vi "GUI_Beampointing2_Pico.vi"() -> ()   [LabVIEW 2013]
uses:
  shared programs/GUI_Template/GUI_master/tcp_new_data_event.ctl
  shared programs/GUI_Template/GUI_master/tcp new data cluster.ctl
  Ctrs/beam detection.ctl
  Ctrs/move_old.ctl
  Ctrs/stats.ctl
  Ctrs/Motor Calibration.ctl
  <vilib>/Analysis/NI_AALBase.lvlib
panel:
  in  "size 2":cluster{"xhair size":dbl, "xhair size 2":dbl}={"xhair size"=20.0, "xhair size 2"=20.0} {"xhair size 2" min=0.0 max=0.0; "xhair size" min=0.0 max=0.0}
  in  "Time":timestamp[](array[timestamp])
  in  "Stats 2":T1
  in  "output cluster 2":T2
  in  "UDP error message":string
  in  "Save Stats":bool
  in  "output cluster":T6={"img to avg"=0, "beam detection para"={"Filter"=0, "Filter Para"={"X Size"=0, "Y Size"=0, "% Tolerance"=0}, "detection method"=0, "smal para"=[], "Remove small Objects"=FALSE, "Restrict to round Objects"=FALSE}, "move"={"Tolerance [%]"=0.1, "Stepsize"=0.0001, "Invert Axis"=TRUE, "Invert Direction X"=FALSE, "Invert Direction Y"=TRUE, "enable feedback"=FALSE, "Set Centriod Target"=FALSE, "my active motor"=""}, "GUIdevice 1"="", "GUIdevice 2"="", "ActiveMotor"=0, "stats path "=path ""} {"beam detection para"."smal para"."Measurement Parameter" items=["Center of Mass X", "Center of Mass Y", "First Pixel X", "First Pixel Y", "Bounding Rect Left", "Bounding Rect Top", "Bounding Rect Right", "Bounding Rect Bottom", "Max Feret Diameter Start X", "Max Feret Diameter Start Y", "Max Feret Diameter End X", "Max Feret Diameter End Y", "Max Horiz. Segment Length Left", "Max Horiz. Segment Length Right", "Max Horiz. Segment Length Row", "-", "Bounding Rect Width", "Bounding Rect Height", "Bounding Rect Diagonal", "Perimeter", "Convex Hull Perimeter", "Holes' Perimeter", "Max Feret Diameter", "Equivalent Ellipse Major Axis", "Equivalent Ellipse Minor Axis", "Equivalent Ellipse Minor Axis (Feret)", "Equivalent Rect Long Side", "Equivalent Rect Short Side", "Equivalent Rect Diagonal", "Equivalent Rect Short Side (Feret)", "Average Horiz. Segment Length", "Average Vert. Segment Length", "Hydraulic Radius", "Waddel Disk Diameter", "-", "Area", "Holes' Area", "Particle & Holes' Area", "Convex Hull Area", "Image Area", "-", "Number of Holes", "Number of Horiz. Segments", "Number of Vert. Segments", "-", "Orientation", "Max Feret Diameter Orientation", "-", "% Area/Image Area", "% Area/(Particle & Holes' Area)", "Ratio of Equivalent Ellipse Axes", "Ratio of Equivalent Rect Sides", "-", "Elongation Factor", "Compactness Factor", "Heywood Circularity Factor", "Type Factor", "-", "Sum X", "Sum Y", "Sum XX", "Sum XY", "Sum YY", "Sum XXX", "Sum XXY", "Sum XYY", "Sum YYY", "-", "Moment of Inertia XX", "Moment of Inertia XY", "Moment of Inertia YY", "Moment of Inertia XXX", "Moment of Inertia XXY", "Moment of Inertia XYY", "Moment of Inertia YYY", "Norm. Moment of Inertia XX", "Norm. Moment of Inertia XY", "Norm. Moment of Inertia YY", "Norm. Moment of Inertia XXX", "Norm. Moment of Inertia XXY", "Norm. Moment of Inertia XYY", "Norm. Moment of Inertia YYY", "Hu Moment 1", "Hu Moment 2", "Hu Moment 3", "Hu Moment 4", "Hu Moment 5", "Hu Moment 6", "Hu Moment 7"]; "beam detection para"."smal para"."Range Lower Value" format="%.2f"; "beam detection para"."smal para"."Range Upper Value" format="%.2f"; "beam detection para"."detection method" items=["clustering", "entropy", "metric", "moments", "inter-class variance"]; "beam detection para"."Filter" items=["No Filter", "Median Filter", "Low Pass Filter"]}
  in  "Trigger::1":bool
  in  "Triggerdelay::1":dbl=0.003 min=0.0 max=0.09 format="%#_6f"
  in  "Exposure::1":dbl=0.095 min=0.0001 max=1.0 format="%#_6f"
  in  "ActiveMotorName::2":string
  in  "RelativeSettings.Axis 1.StepSize::2":dbl=50.0 caption="Axis 1 Stepsize" min=0.0 max=999999.0 format="%_4p"
  in  "RelativeSettings.Axis 2.StepSize::2":dbl=50.0 caption="Axis 2 StepSize" min=0.0 max=999999.0 format="%_4p"
  in  "RelativeSettings.Axis 2.Position::2":dbl caption="Axis 2 Position" min=-999999.0 max=999999.0 format="%_4p"
  in  "RelativeSettings.Axis 1.Position::2":dbl caption="Axis 1 Position" min=-999999.0 max=999999.0 format="%_4p"
  in  "RelativeMove.Axis 2.CW::2":bool caption="RelativeMove.Axis 2.CW::1"
  in  "RelativeMove.Axis 2.CCW::2":bool caption="RelativeMove.Axis. 2.CCW::1"
  in  "RelativeMove.Axis 1.CW::2":bool caption="RelativeMove.Axis 1.CW::1"
  in  "RelativeMove.Axis 1.CCW::2":bool caption="RelativeMove.Axis 1.CCW::1"
  out "Names":string[](array[string])=["PA2_Input1", "PA2_Input2", "L2_TelInpFar", "L1_TelInpNear", "L4_TREXPASS1", "L5_TREXPass2", "L6_TREXPass3", "L7_TREXPass4", "L8_M10Leak", "B1_TelInput", "B2_TelLens1"]
  in  "ActiveMotor":u16(ring)=7
  in  "Set Centriod Target":bool
  in  "size":dbl=10.299999999999997
  in  "Tab Control 2":enum32{"CCD Original ", "CCD Detected"}(tab)=enum."CCD Detected"
  out "image::1":T7(plugin-control) caption="StagingM1Far"
  out "Beam":T7(plugin-control)
  in  "Reset History":bool
  out "centriod X":dbl[](graph)=[249.59745762711864, 249.9873417721519, 249.85593220338984]
  out "centriod Y":dbl[](graph)=[256.39830508474574, 256.0126582278481, 257.0]
  out "Stats":cluster{timestamp[], dbl[]}[](graph)
  in  "Tab Control":enum32{"System", "Detection", "Feedback"}(tab)=enum."Feedback"
  in  "Save Stats":bool
  in  "update speed [ms]":i32=200
  in  "img to avg":i32=20
  in  "Save Config":bool
  in  "Load Config":bool
  in  "Cameras":u16(ring)=15 items=["10TW_Driver_Spot_Cam", "B1_TelInput", "B2_TelLens1", "B3_TelLens2", "B5_CompressorOut", "B6_SwitchYNear", "B9_OAPFront", "GIGEtest", "L1_TelInpNear", "L2_TelInpFar", "L3_TelescopeOut", "L4_TREXpass1", "L5_TREXPass2", "L6_TREXpass3", "L7_TREXPass4", "L8_M10Leak", "OAPtestCam", "PA2_Input1", "PA2_Input2", "PaperCam", "StagingAlignBeam1", "StagingAlignBeam2", "StagingCapAlignment", "StagingCapSpec", "StagingCapSpec1stOrder", "StagingChromaxGuppy", "StagingDiodeMonitor", "StagingFocusBeam1", "StagingFocusBeam2", "StagingGuppy", "StagingM1Far", "StagingM1Near", "StagingM3Far", "StagingM4", "StagingM5", "StagingMagnetCam1", "StagingMagnetCam2", "StagingMagnetCam3", "StagingManta2", "StagingModeImager2", "StagingModeTemp", "StagingOAP1Far", "StagingOAP1Near", "StagingOAP2Far", "StagingOAP2Near", "StagingPhasics", "StagingPhosphor", "StagingTapeCam", "StagingTapeMonitorCam", "StagingTopView", "TargetCam10Hz_Diode", "TargetCam1Hz_Pulsed", "TREXVarianCam0", "TREXVarianCam1", "TREXVarianCam2", "TREXVarianCam3", "TREX_CapSideView", "TREX_TA6", "TS-253a_in", "TS-CapSideview", "TS-CapSpec", "TS-ChromexCam", "TS-InputNearField", "TS-Mode1", "TS-OverlapCam", "TS-Periscope", "XUV_Cam1", "XUV_Cam2"]
  in  "calibrate":bool
  in  "stats path":path
  in  "beam detection para":T3={"Filter"=1, "Filter Para"={"X Size"=5, "Y Size"=5, "% Tolerance"=1}, "detection method"=4, "smal para"=[{"Measurement Parameter"=35, "Range Lower Value"=150.0, "Range Upper Value"=300.0, "Range"=FALSE, "Measurement Type"=FALSE}], "Remove small Objects"=TRUE, "Restrict to round Objects"=FALSE} {"smal para"."Measurement Parameter" items=["Center of Mass X", "Center of Mass Y", "First Pixel X", "First Pixel Y", "Bounding Rect Left", "Bounding Rect Top", "Bounding Rect Right", "Bounding Rect Bottom", "Max Feret Diameter Start X", "Max Feret Diameter Start Y", "Max Feret Diameter End X", "Max Feret Diameter End Y", "Max Horiz. Segment Length Left", "Max Horiz. Segment Length Right", "Max Horiz. Segment Length Row", "-", "Bounding Rect Width", "Bounding Rect Height", "Bounding Rect Diagonal", "Perimeter", "Convex Hull Perimeter", "Holes' Perimeter", "Max Feret Diameter", "Equivalent Ellipse Major Axis", "Equivalent Ellipse Minor Axis", "Equivalent Ellipse Minor Axis (Feret)", "Equivalent Rect Long Side", "Equivalent Rect Short Side", "Equivalent Rect Diagonal", "Equivalent Rect Short Side (Feret)", "Average Horiz. Segment Length", "Average Vert. Segment Length", "Hydraulic Radius", "Waddel Disk Diameter", "-", "Area", "Holes' Area", "Particle & Holes' Area", "Convex Hull Area", "Image Area", "-", "Number of Holes", "Number of Horiz. Segments", "Number of Vert. Segments", "-", "Orientation", "Max Feret Diameter Orientation", "-", "% Area/Image Area", "% Area/(Particle & Holes' Area)", "Ratio of Equivalent Ellipse Axes", "Ratio of Equivalent Rect Sides", "-", "Elongation Factor", "Compactness Factor", "Heywood Circularity Factor", "Type Factor", "-", "Sum X", "Sum Y", "Sum XX", "Sum XY", "Sum YY", "Sum XXX", "Sum XXY", "Sum XYY", "Sum YYY", "-", "Moment of Inertia XX", "Moment of Inertia XY", "Moment of Inertia YY", "Moment of Inertia XXX", "Moment of Inertia XXY", "Moment of Inertia XYY", "Moment of Inertia YYY", "Norm. Moment of Inertia XX", "Norm. Moment of Inertia XY", "Norm. Moment of Inertia YY", "Norm. Moment of Inertia XXX", "Norm. Moment of Inertia XXY", "Norm. Moment of Inertia XYY", "Norm. Moment of Inertia YYY", "Hu Moment 1", "Hu Moment 2", "Hu Moment 3", "Hu Moment 4", "Hu Moment 5", "Hu Moment 6", "Hu Moment 7"]; "smal para"."Range Lower Value" format="%.2f"; "smal para"."Range Upper Value" format="%.2f"; "detection method" items=["clustering", "entropy", "metric", "moments", "inter-class variance"]; "Filter" items=["No Filter", "Median Filter", "Low Pass Filter"]}
  in  "Move Properties":T5={"Tolerance [%]"=0.1, "Stepsize"=0.0001, "Invert Axis"=TRUE, "Invert Direction X"=FALSE, "Invert Direction Y"=TRUE, "enable feedback"=FALSE, "Set Centriod Target"=FALSE, "my active motor"=""} {"Stepsize" format="%#_6p"}
  out "Y Size":dbl=20.599999999999994
  out "X Size":dbl=15.599999999999994
  out "Particle Reports (Pixels)":T8(array[cluster])=[{"Area"=236.0, "Number of Holes"=0.0, "Bounding Rect"={"Left"=243.0, "Top"=247.0, "Right"=258.0, "Bottom"=268.0}, "Center of Mass"={"X"=249.85593220338984, "Y"=257.0}, "Orientation"=87.89795034558499, "Dimensions"={"Width"=15.0, "Height"=21.0}}] {"Orientation" format="%.2f"; "Dimensions"."Height" format="%.2f"; "Dimensions"."Width" format="%.2f"; "Center of Mass"."Y" format="%.2f"; "Center of Mass"."X" format="%.2f"; "Bounding Rect"."Bottom" format="%.2f"; "Bounding Rect"."Right" format="%.2f"; "Bounding Rect"."Top" format="%.2f"; "Bounding Rect"."Left" format="%.2f"; "Number of Holes" format="%.2f"; "Area" format="%.2f"}
  out "move required":bool=TRUE
  out "moving":bool
  out "Best Rectangle":T9(array[cluster])=[{"Left"=243.0, "Top"=247.0, "Right"=259.0, "Bottom"=267.0}, {"Left"=242.0, "Top"=246.0, "Right"=257.0, "Bottom"=267.0}, {"Left"=242.0, "Top"=246.0, "Right"=258.0, "Bottom"=267.0}, {"Left"=243.0, "Top"=247.0, "Right"=258.0, "Bottom"=268.0}, {"Left"=242.0, "Top"=247.0, "Right"=258.0, "Bottom"=267.0}]
  out "XY Graph":cluster{timestamp[], dbl[]}[](graph)
  out "Y offset":dbl=-1.5635377104373447
  out "X offset":dbl=10.405838585398385
  in  "Target.X::1":dbl=260.0 min=0.0 max=2000.0 format="%#_6f"
  in  "Target.Y::1":dbl=255.0 min=0.0 max=2000.0 format="%#_6f"
  out "mean Y":dbl=256.56353771043734 format="%0.2f"
  out "mean X":dbl=249.59416141460161 format="%0.2f"
  out "beam detected":bool=TRUE
  in  "GUIdevice 2":string="Picopad4"
  out "error out":errorcluster
  in  "insert tag":bool=TRUE
  in  "stop":bool=TRUE
  in  "GUIdevice 1":string="B5_CompressorOut"
  out "tcp data event":T10
  out "error IO 2":errorcluster
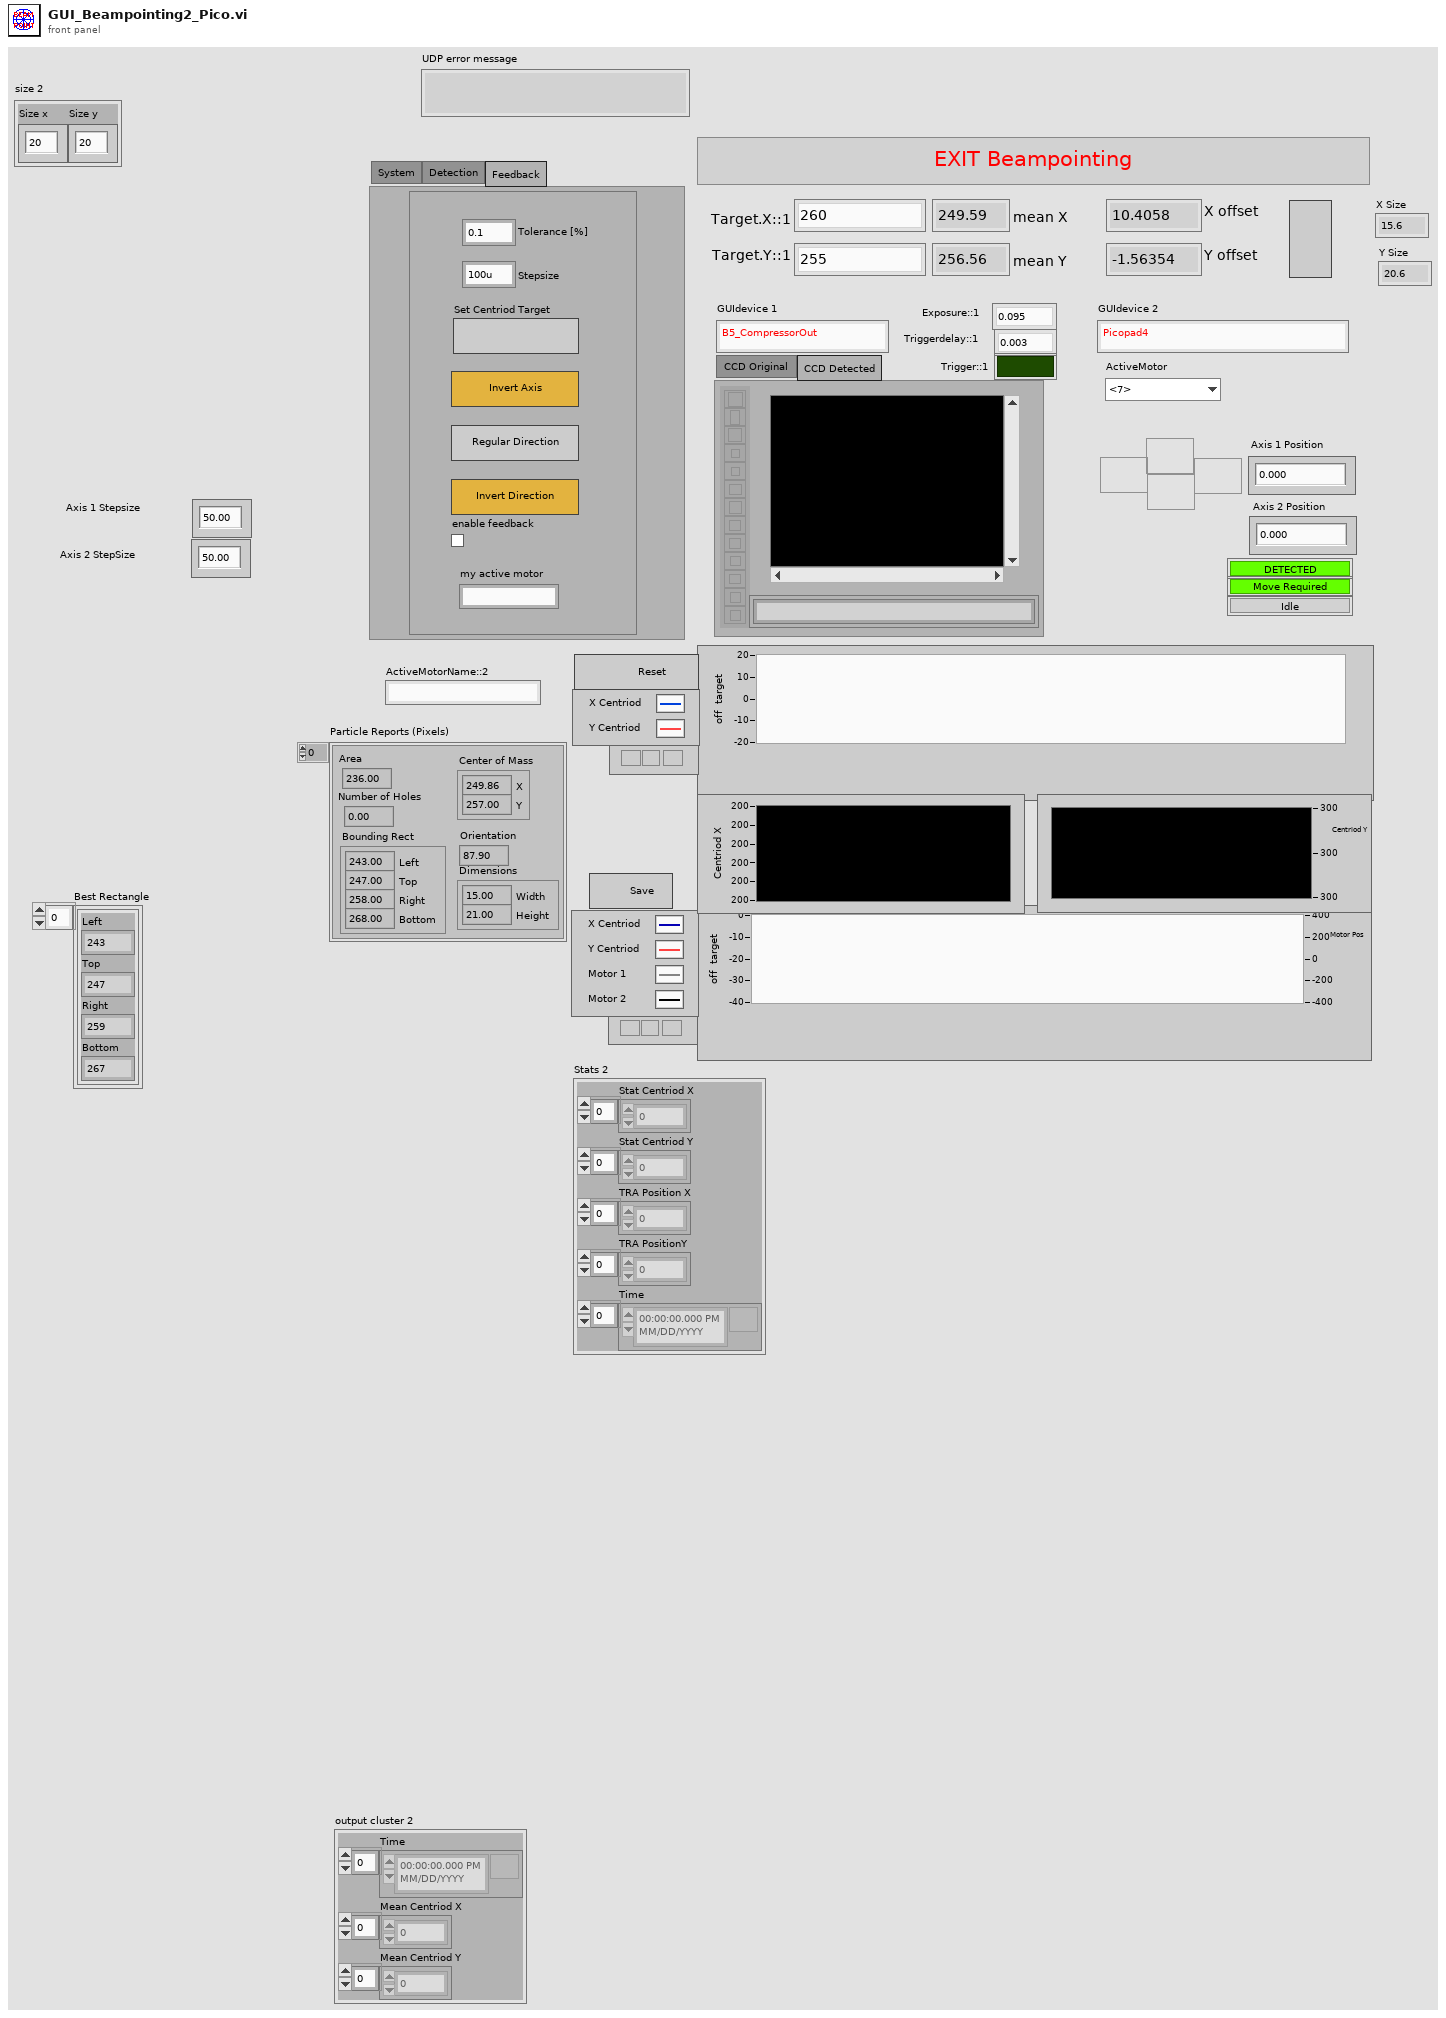
[diagram p1: front panel]
types:
  T1 = typedef "stats.ctl" = cluster{"Stat Centriod X":dbl[], "Stat Centriod Y":dbl[], "TRA Position X":dbl[], "TRA PositionY":dbl[], "Time":timestamp[]}
  T2 = cluster{"Time":timestamp[], "Mean Centriod X":dbl[], "Mean Centriod Y":dbl[]}
  T3 = typedef "beam detection.ctl" = cluster{"Filter":u16, "Filter Para":cluster{"X Size":i32, "Y Size":i32, "% Tolerance":i32}, "detection method":i32, "smal para":cluster{"Measurement Parameter":T4, "Range Lower Value":dbl, "Range Upper Value":dbl, "Range":bool, "Measurement Type":bool}[], "Remove small Objects":bool, "Restrict to round Objects":bool}
  T4 = typedef "Particle Parameters" = i32
  T5 = typedef "move_old.ctl" = cluster{"Tolerance [%]":dbl, "Stepsize":dbl, "Invert Axis":bool, "Invert Direction X":bool, "Invert Direction Y":bool, "enable feedback":bool, "Set Centriod Target":bool, "my active motor":string}
  T6 = cluster{"img to avg":i32, "beam detection para":T3, "move":T5, "GUIdevice 1":string, "GUIdevice 2":string, "ActiveMotor":u16, "stats path ":path}
  T7 = typedef "IMAQ Image.ctl" = refnum<image>
  T8 = cluster{"Area":dbl, "Number of Holes":dbl, "Bounding Rect":cluster{"Left":dbl, "Top":dbl, "Right":dbl, "Bottom":dbl}, "Center of Mass":cluster{"X":dbl, "Y":dbl}, "Orientation":dbl, "Dimensions":cluster{"Width":dbl, "Height":dbl}}[]
  T9 = cluster{"Left":dbl, "Top":dbl, "Right":dbl, "Bottom":dbl}[]
  T10 = typedef "tcp_new_data_event.ctl" = refnum<user-event>
  T11 = typedef "tcp new data cluster.ctl" = cluster{"EventEnum":enum16{"new data", "connection status update"}, "Device name":string}
  T12 = typedef "Image Type" = u32
  T13 = cluster{"RelativeMove.Axis 1.CW::2":refnum<vi>, "RelativeMove.Axis 1.CCW::2":refnum<vi>, "RelativeMove.Axis 2.CW::2":refnum<vi>, "RelativeMove.Axis 2.CCW::2":refnum<vi>}
  T14 = cluster{"Left":i32, "Top":i32, "Right":i32, "Bottom":i32}
  T15 = enum32{"invalid app kind", "Development System", "Run Time System", "Student Edition", "Embedded LabVIEW", "Evaluation", "Custom"}
  T16 = enum32{"Invalid", "Standard", "Closed", "Hidden", "Minimized", "Maximized"}
  T17 = enum16{"open", "replace", "create", "open or create", "replace or create", "replace or create with confirmation"}
  T18 = typedef "Motor Calibration.ctl" = cluster{"Slope Axis 1":dbl, "Axis Inverted":bool, "Slope Axis 2":dbl, "Axis 1 revered":bool, "Axis 2 revered":bool}
  T19 = cluster{"Core":cluster{"Current VI Reference":refnum<vi>, "Close Panel on Exit?":bool}, "beam detection para":T3, "Centriod X":dbl[], "Centriod Y":dbl[], "Best Rectangle":cluster{"Left":dbl, "Top":dbl, "Right":dbl, "Bottom":dbl}[], "PArticle Report":cluster{"Area":dbl, "Number of Holes":dbl, "Bounding Rect":cluster{"Left":dbl, "Top":dbl, "Right":dbl, "Bottom":dbl}, "Center of Mass":cluster{"X":dbl, "Y":dbl}, "Orientation":dbl, "Dimensions":cluster{"Width":dbl, "Height":dbl}}[], "Mean Centriod X":dbl[], "Mean Centriod Y":dbl[], "Time":timestamp[], "beam detected":bool, "offsets":cluster{"X offset":dbl, "Y offset":dbl}, "move":T5, "moving":bool, "Stats":T1, "set centriod target":bool, "Motor Calibration":T18}
  T20 = cluster{"Left":dbl, "Top":dbl, "Right":dbl, "Bottom":dbl}
  T21 = cluster{"Current VI Reference":refnum<vi>, "Close Panel on Exit?":bool}
  T22 = cluster{"Time":timestamp[], "Stat Centriod X":dbl[]}
  T23 = cluster{"Time":timestamp[], "Stat Centriod Y":dbl[]}
  T24 = cluster{"Time":timestamp[], "TRA Position X":dbl[]}
  T25 = cluster{"Time":timestamp[], "TRA PositionY":dbl[]}
  T26 = cluster{"Time":timestamp[], "TRA PositionY":dbl[]}[]
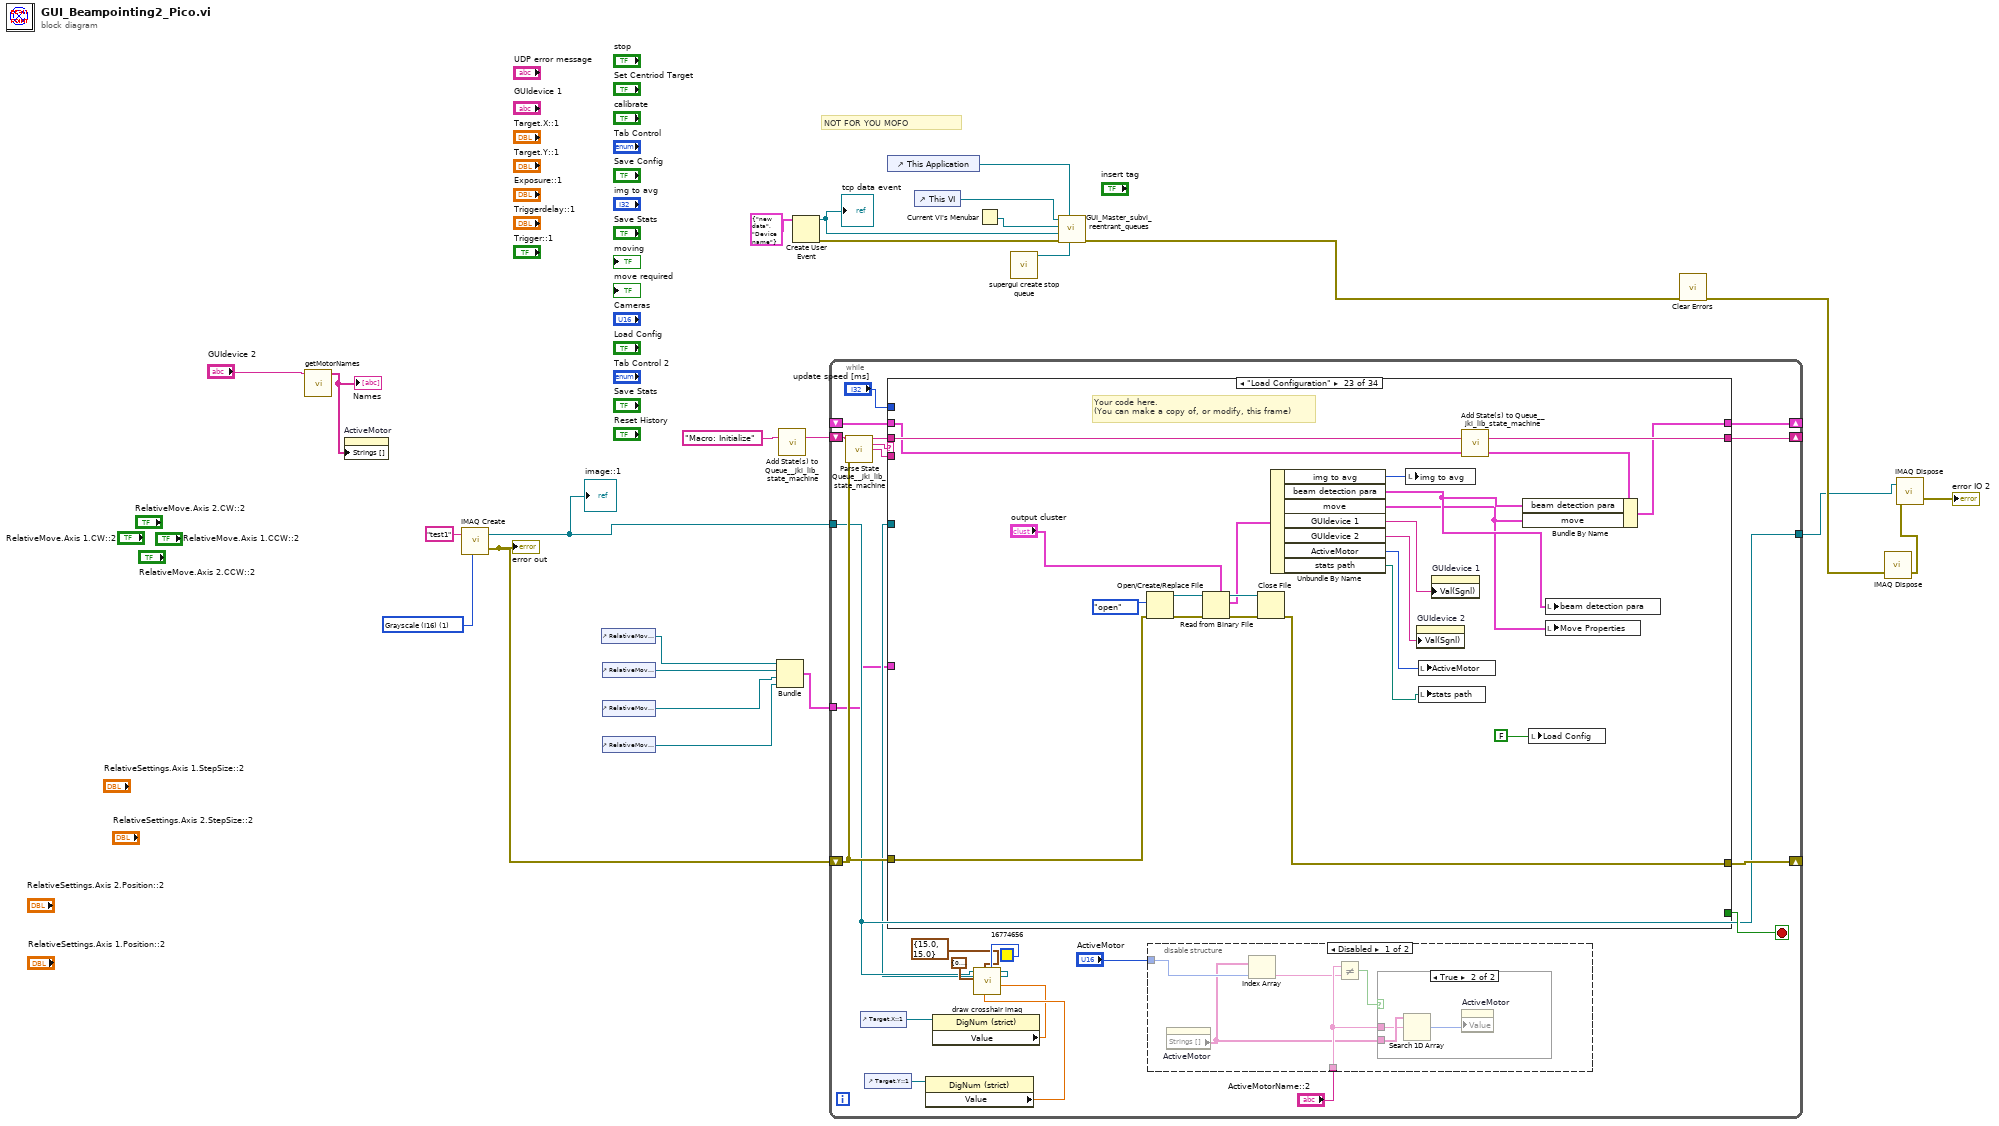
[diagram p0: block diagram]
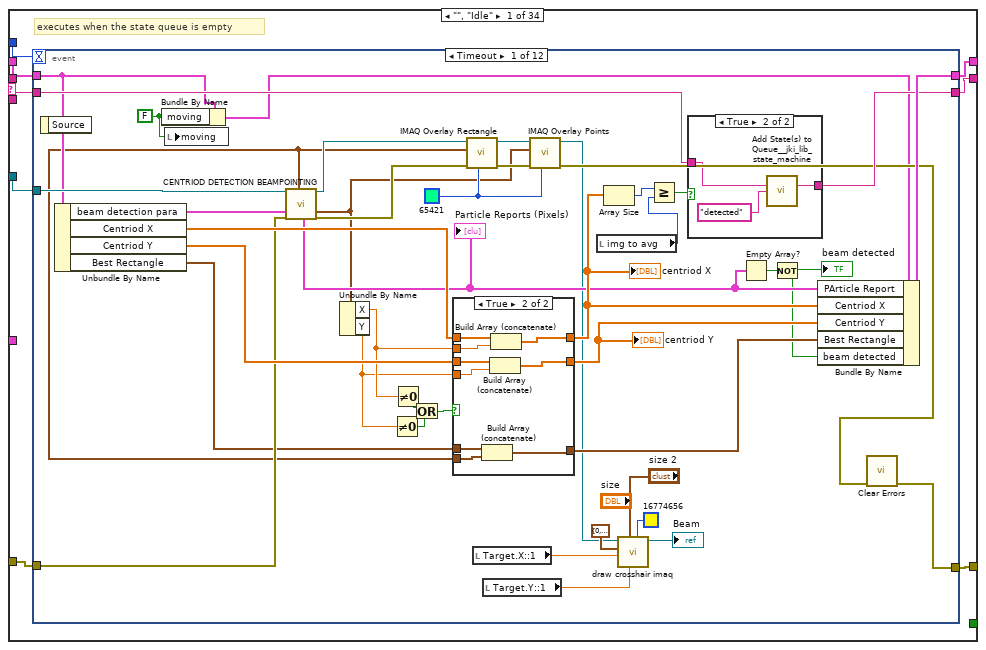
[diagram p4: hidden frame]
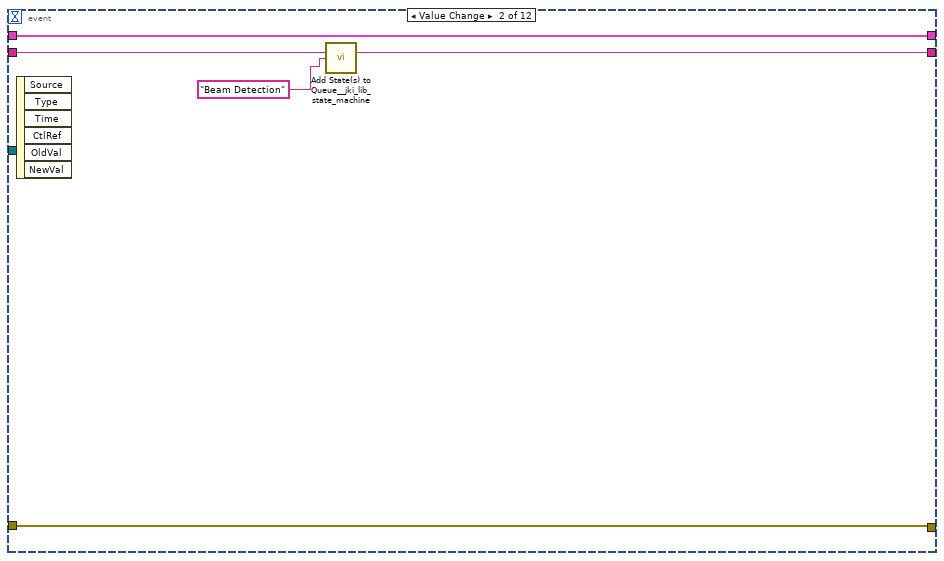
[diagram p7: hidden frame]
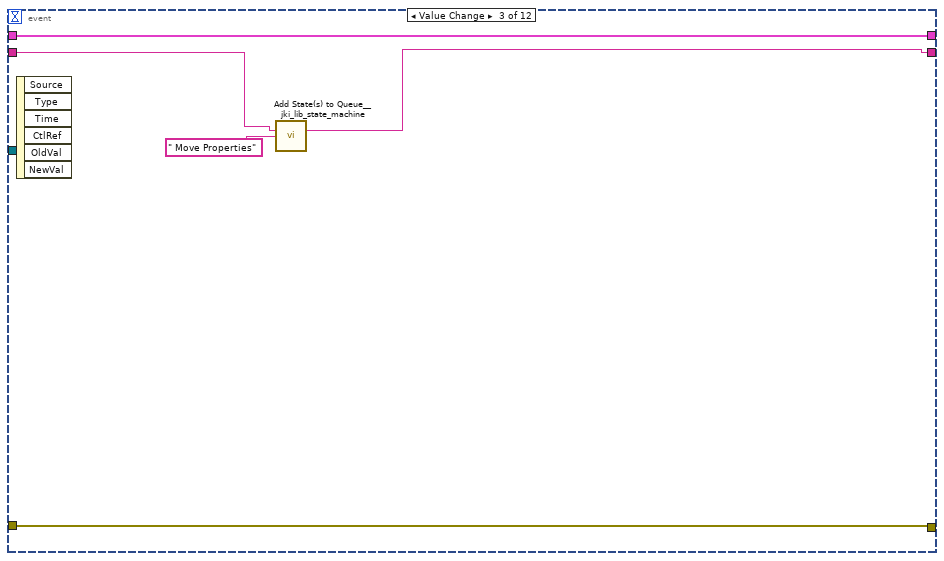
[diagram p8: hidden frame]
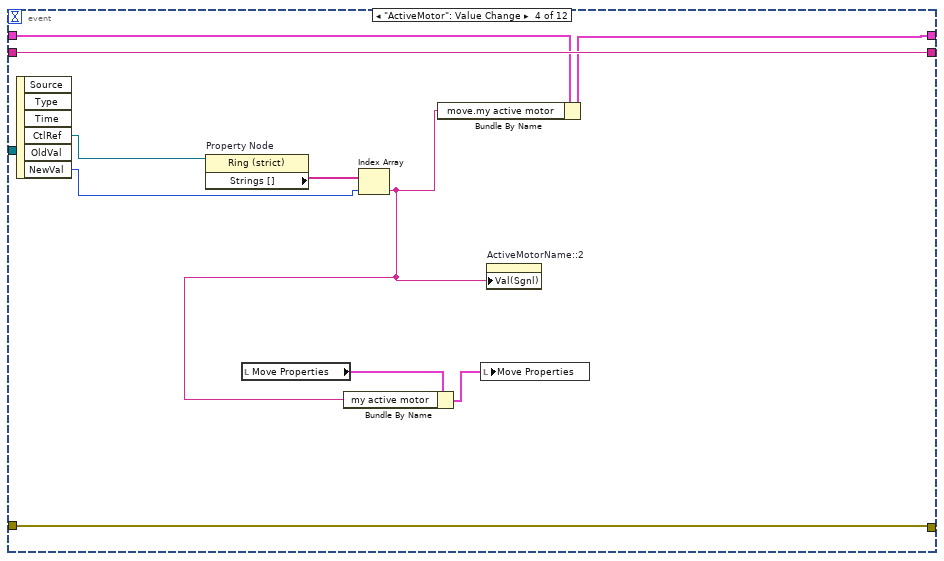
[diagram p9: hidden frame]
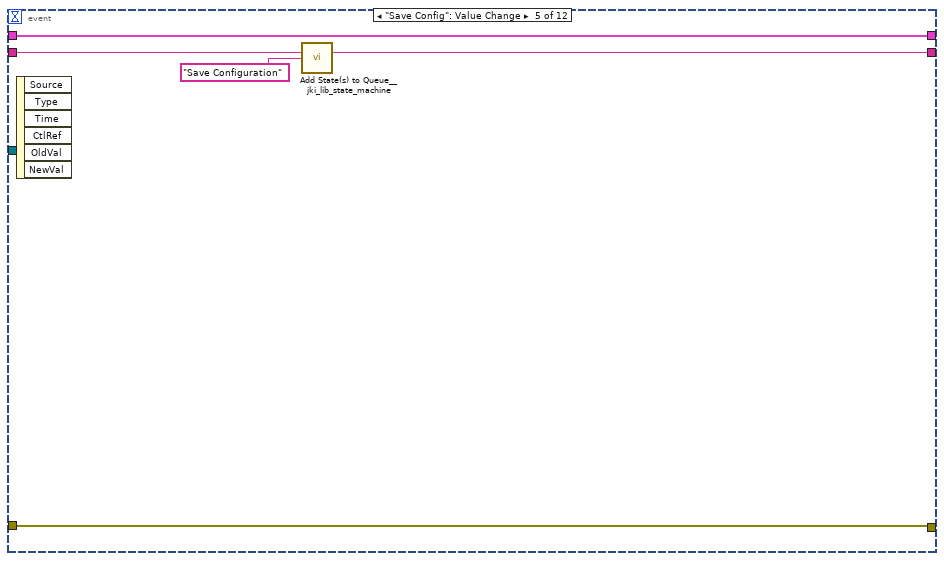
[diagram p10: hidden frame]
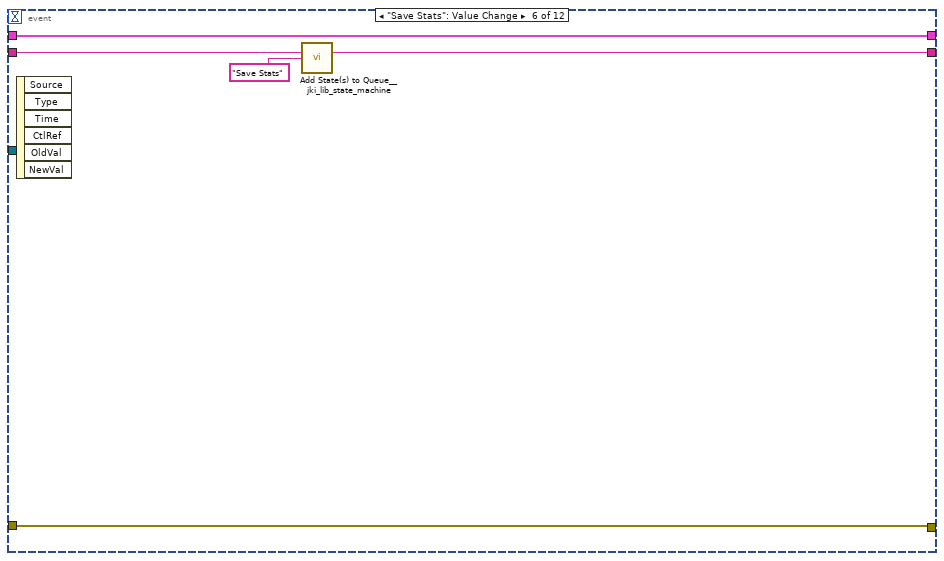
[diagram p11: hidden frame]
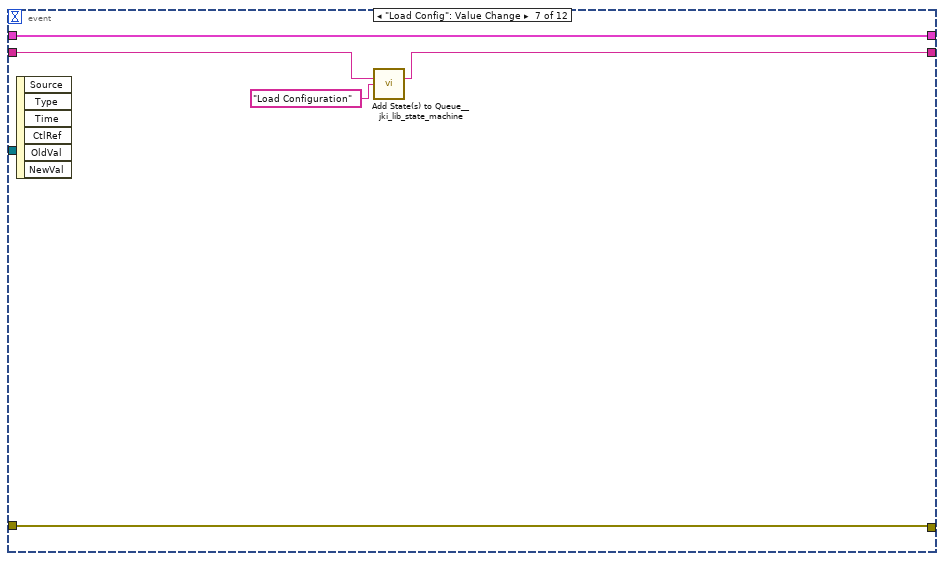
[diagram p12: hidden frame]
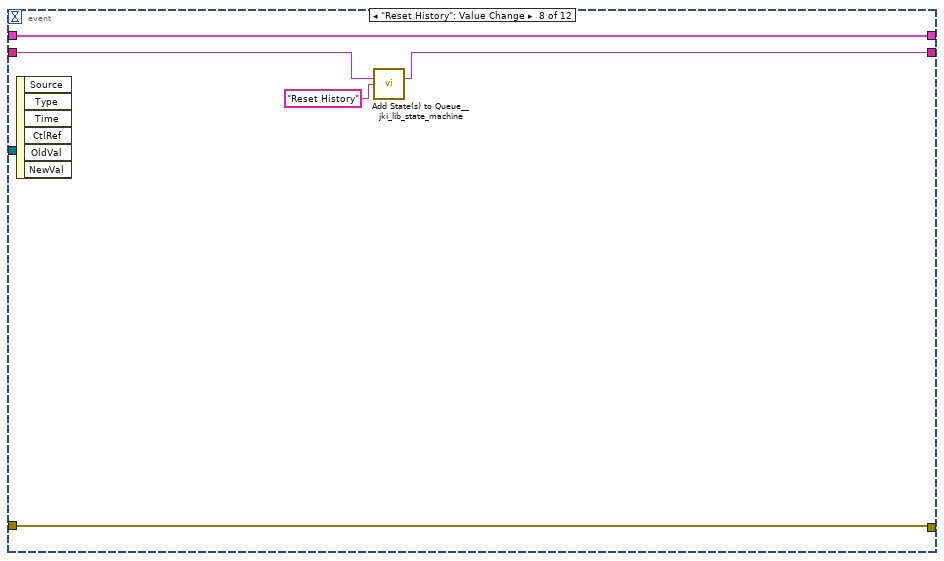
[diagram p13: hidden frame]
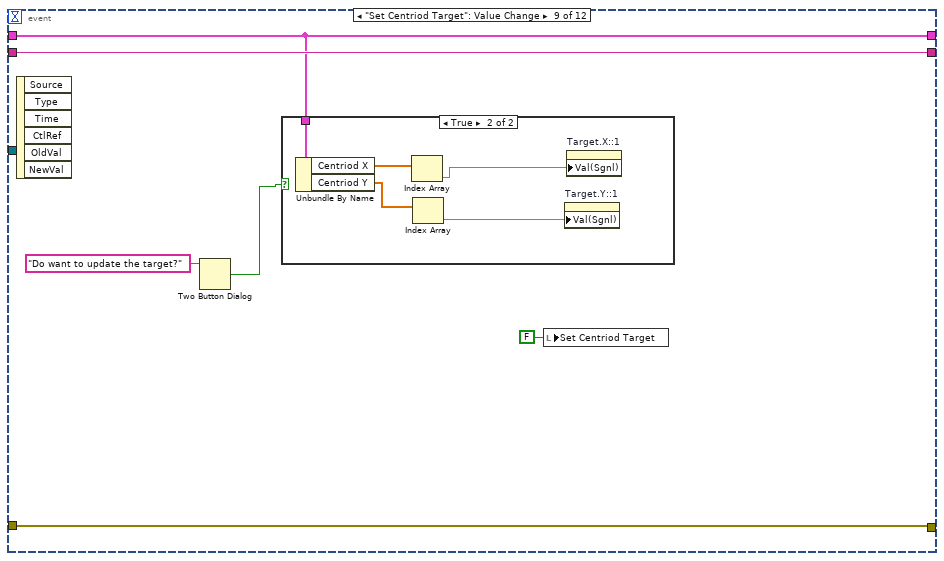
[diagram p14: hidden frame]
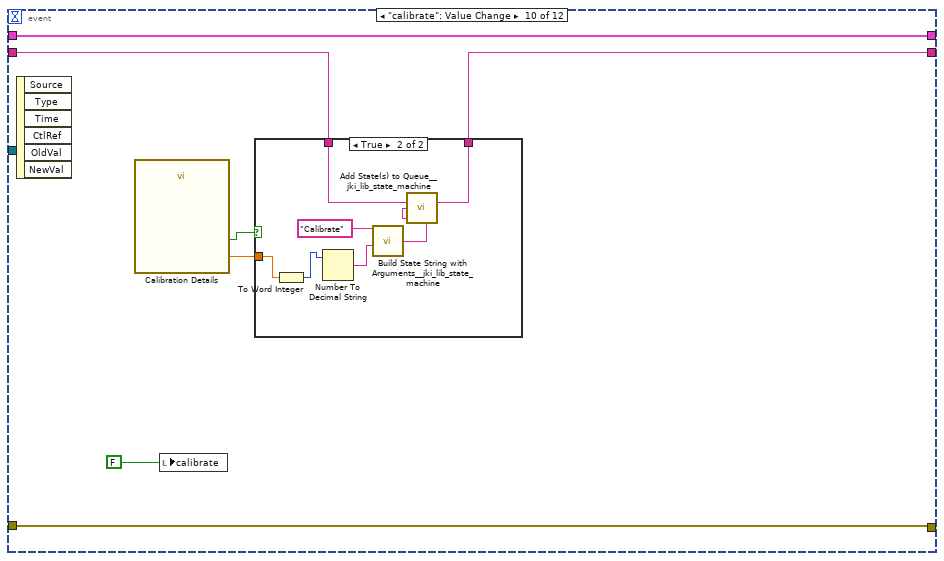
[diagram p16: hidden frame]
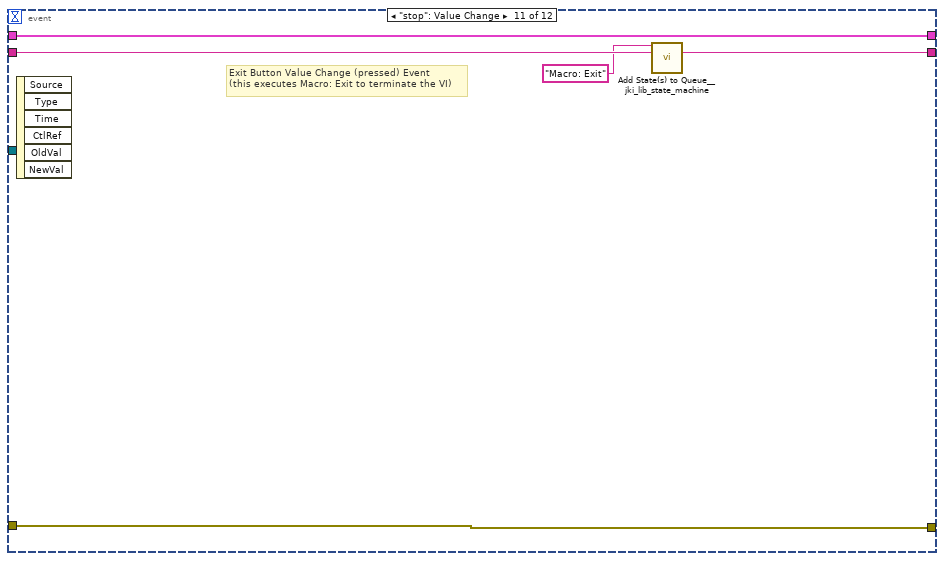
[diagram p18: hidden frame]
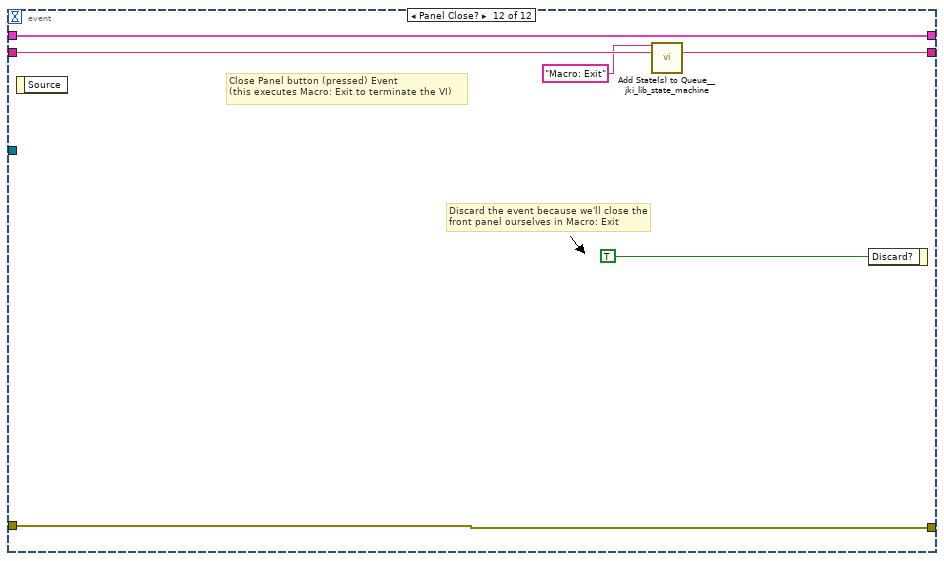
[diagram p19: hidden frame]
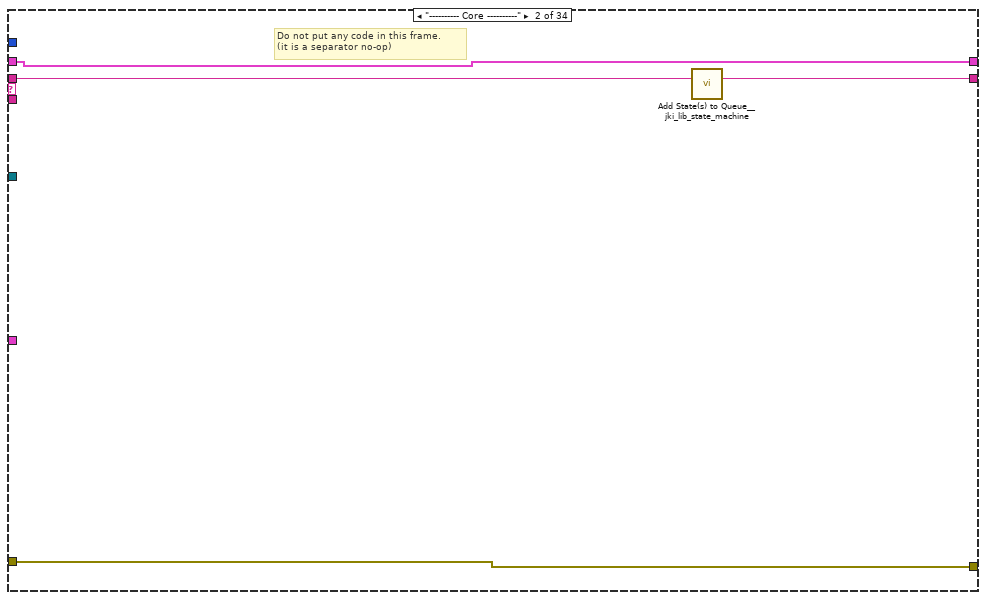
[diagram p20: hidden frame]
diagram:
  w24 = T12 1 items=["Grayscale (U8)", "Grayscale (I16)", "Grayscale (SGL)", "Complex (CSG)", "RGB (U32)", "HSL (U32)", "RGB (U64)", "Grayscale (U16)"] ("Image Type")
  # "NOT FOR YOU MOFO"
  n1 = call "getMotorNames.vi"("DeviceName"="GUIdevice 2") -> ("elements"=w7:string[])  [unwired: 10 in]
  "Names" <- w7
  n2 = property on="ActiveMotor" class="Ring (strict)"("Strings []"=w7) -> ()  [unwired: 2 in, 2 out]
  n3 = call "IMAQ Create"("Image Name"="test1", "Image Type"=w24) -> ("New Image"=w9:T7, "error out"=w17:errorcluster)  [unwired: 3 in]
  "error out" <- w17
  "image::1" <- w9
  n4 = control-ref of="RelativeMove.Axis 1.CW::2"() -> (w6:refnum<vi>)
  n5 = control-ref of="RelativeMove.Axis 1.CCW::2"() -> (w5:refnum<vi>)
  n6 = control-ref of="RelativeMove.Axis 2.CW::2"() -> (w4:refnum<vi>)
  n7 = control-ref of="RelativeMove.Axis 2.CCW::2"() -> (w3:refnum<vi>)
  n8 = Bundle("RelativeMove.Axis 1.CW::2"=w6, "RelativeMove.Axis 1.CCW::2"=w5, "RelativeMove.Axis 2.CW::2"=w4, "RelativeMove.Axis 2.CCW::2"=w3) -> (w2:T13)  [unwired: 1 in]
  n9 = call <vilib>:"Add State(s) to Queue__jki_lib_state_machine.vi"("State(s) in (\"\")"="Macro: Initialize") -> ("States Out"=w19:string)  [unwired: 14 in]
  n10 = Create User Event(user event datatype=T11 {"EventEnum"=enum."new data", "Device name"="Device name"} ("New Event")) -> (user event=w10:refnum<user-event>, error out=w12:errorcluster)  [unwired: 1 in]
  "tcp data event" <- w10
  n11 = while "JKI - String-Based Queued State Machine (Basic) v1.0" {
    shift-right: [w42] -> _
    shift-left: _ -> [w41]
    shift-right: [w44] -> _
    shift-left: w17 -> [w39]
    shift-right: [w43] -> _
    shift-left: w19 -> [w45]
    tunnel: w9 -> [w31]
    tunnel: [w31] -> w16
    tunnel: w2 -> [w29]
    stop <- w38 stop-if-true
    n12 = call <vilib>:"Parse State Queue__jki_lib_state_machine.vi"("State Queue"=w45, "Error In (no error)"=w39) -> ("Remaining States"=w47:string, "Current State"=w48:string, "Arguments"=w46:string)  [unwired: 11 in]
    n13 = control-ref of="Target.X::1"() -> (w34:refnum<vi>)
    n14 = control-ref of="Target.Y::1"() -> (w35:refnum<vi>)
    n15 = property class="DigNum (strict)"(reference=w35) -> ("Value"=w37:dbl)  [unwired: 1 in, 2 out]
    n16 = property class="DigNum (strict)"(reference=w34) -> ("Value"=w36:dbl)  [unwired: 1 in, 2 out]
    n17 = call "draw crosshair imaq.vi"("Color"=u32 16774656, "Target.Y"=w37, "size"=cluster{"xhair size":dbl, "xhair size 2":dbl} {"xhair size"=15.0, "xhair size 2"=15.0}, "Target.X"=w36, "Bounding Rectangle"=T14 {"Left"=0, "Top"=0, "Right"=0, "Bottom"=0}, "image in"=w31) -> ("image out"=w30:T7)  [unwired: 4 in, 1 out]
    n18 = case shown="\"Load Configuration\"" w48 {
      selector: w48 -> [_ _ w204 _ _ _ _ _ _ _ _ _ _ _ _ _ _ _ _ _ _ _ _ _ _ _ _ _ _ _ _ _ _ _]
      tunnel: w47 -> [w64 w203 w208 w226 w232 w237 w241 w265 w271 w275 w279 w285 w296 w322 w327 w337 w341 w347 w354 w375 w383 w404 w440 w448 w452 w485 w495 w532 w556 w628 w688 w701 w776 w780]
      tunnel: w46 -> [_ _ _ _ _ _ _ _ _ _ _ w280 w290 _ _ _ _ _ _ _ _ _ _ _ _ _ _ _ _ _ _ w694 w771 _]
      tunnel: w41 -> [w62 w200 w206 w217 w229 w235 w238 _ w267 w272 w277 w283 w292 w319 w324 w334 w338 w343 w350 w358 w381 w402 w432 w444 w449 w468 w497 w529 w543 w615 w684 w723 w773 w777]
      tunnel: [w61 w201 w210 w223 errorcluster {"status"=FALSE, "code"=0, "source"=""} ("error out") w234 w239 w262 w268 w273 w276 w281 w293 w320 w325 w335 w339 w345 w352 w363 w379 w400 w429 w446 w450 w484 w516 w530 w554 w626 w677 w725 w772 w778] -> w44
      tunnel: w39 -> [w60 w201 w209 w223 w228 w234 w239 w262 w269 w273 w276 w282 w294 w320 w325 w335 w339 w345 w352 w364 w380 w401 w430 w446 w450 w484 w516 w530 w554 w626 w678 w725 w772 w778]
      tunnel: [w63 w202 w207 w225 w231 w236 w240 w264 w270 w274 w278 w284 w295 w321 w326 w336 w340 w346 w353 w374 w382 w403 w439 w447 w451 w453 w503 w531 w555 w627 w687 w726 w775 w779] -> w43
      tunnel: [_ _ _ _ _ TRUE _ _ _ _ _ _ _ _ _ _ _ _ _ _ _ _ _ _ _ _ _ _ _ _ _ _ _ _] -> w38
      tunnel: [w59 w200 w206 w224 w229 w235 w238 w263 w267 w272 w277 w283 w292 w319 w324 w334 w338 w342 w349 w358 w381 w402 w431 w443 w449 w467 w501 w529 w553 w625 w685 w713 w773 w777] -> w42
      tunnel: "update speed [ms]" -> [w58 _ _ _ _ _ _ _ _ _ _ _ _ _ _ _ _ _ _ _ _ _ _ _ _ _ _ _ _ _ _ _ _ _]
      tunnel: w30 -> [w57 _ _ _ _ _ _ _ _ _ _ _ _ _ _ _ _ _ _ _ _ _ _ _ _ _ _ _ _ _ _ _ w770 _]
      tunnel: w29 -> [_ _ _ _ _ _ _ _ _ _ _ _ _ _ _ _ _ _ _ _ _ _ _ _ _ _ _ _ w548 w620 _ _ w774 _]
      frame "", "Idle" {
        # "executes when the state queue is empty"
        n19 = event shown="[0] Timeout" {
          selector: _ -> [_ _ _ _ _ _ _ _ _ _ _ _]
          dyn-events: _ -> [_ _ _ _ _ _ _ _ _ _ _ _]
          timeout: w58 -> [_ _ _ _ _ _ _ _ _ _ _ _]
          tunnel: w64 -> [w86 w126 w131 w138 w146 w151 w155 w160 w167 w177 w193 w199]
          tunnel: [w85 w125 w129 w138 w144 w149 w154 w159 w167 w176 w192 w198] -> w63
          tunnel: w62 -> [w76 w127 w132 w137 w147 w152 w157 w162 w166 w179 w190 w196]
          tunnel: [w82 w124 w128 w139 w143 w148 w156 w161 w168 w180 w191 w197] -> w61
          tunnel: w60 -> [w101 w124 w128 w139 w143 w148 w156 w161 w168 w180 w191 w197]
          tunnel: [w104 w127 w132 w136 w147 w152 w157 w162 w166 w179 w190 w196] -> w59
          tunnel: w57 -> [w105 _ _ _ _ _ _ _ _ _ _ _]
          event Timeout {
            w74 = FALSE ("moving")
            w93 = u32 65421 ("Color")
            n20 = event-data() -> ()  [unwired: 1 in, 1 out]
            n21 = Unbundle By Name(w76) -> ("beam detection para"=w106:T3, "Centriod X"=w103:dbl[], "Centriod Y"=w102:dbl[], "Best Rectangle"=w95:T9)
            n22 = Bundle By Name(cluster=w76, "moving"=w74) -> (w75:T19)
            n23 = local write "moving"(w74) -> ()
            n24 = call "CENTRIOD DETECTION BEAMPOINTING.vi"("Refnum in"=w105, "beam detection para"=w106, "error in (no error)"=w101) -> ("Bounding Rect"=w66:T20, "Particle Reports (Pixels)"=w79:T8, "Refnum out"=w90:T7, "Centriod"=w67:cluster{"X":dbl, "Y":dbl}, "error out"=w84:errorcluster)  [unwired: 10 in, 2 out]
            "Particle Reports (Pixels)" <- w79
            n25 = Unbundle By Name(w67) -> ("X"=w98:dbl, "Y"=w97:dbl)
            n26 = Not Equal To 0?(x=w97) -> (x != 0?=w100:bool)
            n27 = Not Equal To 0?(x=w98) -> (x != 0?=w99:bool)
            n28 = Or(x=w99, y=w100) -> (x .or. y?=w96:bool)
            n29 = case shown="True" w96 {
              tunnel: w103 -> [w113 w122]
              tunnel: w102 -> [w112 w121]
              tunnel: [w113 w120] -> w88
              tunnel: [w112 w119] -> w89
              tunnel: w98 -> [_ w118]
              tunnel: w97 -> [_ w117]
              tunnel: w95 -> [w111 w116]
              tunnel: w66 -> [_ w115]
              tunnel: [w111 w114] -> w94
              frame False {
              }
              frame True {
                n30 = Build Array (concatenate)(w116, w115) -> (w114:T9)
                n31 = Build Array (concatenate)(w121, w117) -> (w119:dbl[])
                n32 = Build Array (concatenate)(w122, w118) -> (w120:dbl[])
              }
            }
            "centriod X" <- w88
            "centriod Y" <- w89
            n33 = call "IMAQ Overlay Rectangle"("Color"=w93, "error in (no error)"=w84, "Rectangle"=w66, "Image"=w90) -> ("error out"=w91:errorcluster, "Image Out"=w92:T7)  [unwired: 6 in]
            n34 = local read "Target.X::1"() -> (w69:dbl)
            n35 = local read "Target.Y::1"() -> (w68:dbl)
            n36 = call "IMAQ Overlay Points"("Color"=w93, "error in (no error)"=w91, "Point"=w67, "Image"=w92) -> ("error out"=w83:errorcluster, "Image Out"=w71:T7)  [unwired: 6 in]
            n37 = local read "img to avg"() -> (w80:i32)
            n38 = Array Size(array=w88) -> (size(s)=w81:i32)
            n39 = call "draw crosshair imaq.vi"("Color"=u32 16774656, "Target.Y"=w68, "size"="size 2", "Target.X"=w69, "Bounding Rectangle"=T14 {"Left"=0, "Top"=0, "Right"=0, "Bottom"=0}, "image in"=w71) -> ("image out"=→"Beam":T7)  [unwired: 4 in, 1 out]
            n40 = Greater Or Equal?(x=w81, y=w80) -> (x >= y?=w87:bool)
            n41 = case shown="True" w87 {
              tunnel: w86 -> [w107 w110]
              tunnel: [w107 w109] -> w85
              frame False {
              }
              frame True {
                n42 = call <vilib>:"Add State(s) to Queue__jki_lib_state_machine.vi"("State(s) in (\"\")"=w110, "State(s) at Back (\"\")"="detected" ("State(s) in Front (\"\")")) -> ("States Out"=w109:string)  [unwired: 13 in]
              }
            }
            n43 = Empty Array?(array=w79) -> (empty?=w78:bool)
            n44 = Not(x=w78) -> (.not. x?=w77:bool)
            "beam detected" <- w77
            n45 = Bundle By Name(cluster=w75, "PArticle Report"=w79, "Centriod X"=w88, "Centriod Y"=w89, "Best Rectangle"=w94, "beam detected"=w77) -> (w104:T19)
            n46 = call <vilib>:"Clear Errors.vi"("error in (no error)"=w83) -> ("error out"=w82:errorcluster)  [unwired: 6 in]
          }
          event Value Change {
            n47 = event-data() -> ()  [unwired: 1 in, 6 out]
            n48 = call <vilib>:"Add State(s) to Queue__jki_lib_state_machine.vi"("State(s) in (\"\")"=w126, "State(s) at Back (\"\")"="Beam Detection" ("State(s) at Back (\"\")")) -> ("States Out"=w125:string)  [unwired: 13 in]
          }
          event Value Change {
            n49 = event-data() -> ()  [unwired: 1 in, 6 out]
            n50 = call <vilib>:"Add State(s) to Queue__jki_lib_state_machine.vi"("State(s) in (\"\")"=w131, "State(s) at Back (\"\")"=" Move Properties" ("State(s) at Back (\"\")")) -> ("States Out"=w129:string)  [unwired: 13 in]
          }
          event "ActiveMotor": Value Change {
            n51 = event-data() -> ("CtlRef"=w141:refnum<vi>, "NewVal"=w140:u16)  [unwired: 1 in, 4 out]
            n52 = property on="Property Node" class="Ring (strict)"(reference=w141) -> ("Strings []"=w142:string[])  [unwired: 1 in, 2 out]
            n53 = local read "Move Properties"() -> (w135:T5)
            n54 = Index Array(array=w142, index=w140) -> (element=w134:string)
            n55 = Bundle By Name(cluster=w135, "my active motor"=w134) -> (w133:T5)
            n56 = Bundle By Name(cluster=w137, "move.my active motor"=w134) -> (w136:T19)
            n57 = local write "Move Properties"(w133) -> ()
            n58 = property on="ActiveMotorName::2" class="Str"("Val(Sgnl)"=w134) -> ()  [unwired: 2 in, 2 out]
          }
          event "Save Config": Value Change {
            n59 = event-data() -> ()  [unwired: 1 in, 6 out]
            n60 = call <vilib>:"Add State(s) to Queue__jki_lib_state_machine.vi"("State(s) in (\"\")"=w146, "State(s) at Back (\"\")"="Save Configuration" ("State(s) in Front (\"\")")) -> ("States Out"=w144:string)  [unwired: 13 in]
          }
          event "Save Stats": Value Change {
            n61 = event-data() -> ()  [unwired: 1 in, 6 out]
            n62 = call <vilib>:"Add State(s) to Queue__jki_lib_state_machine.vi"("State(s) in (\"\")"=w151, "State(s) at Back (\"\")"="Save Stats" ("State(s) in Front (\"\")")) -> ("States Out"=w149:string)  [unwired: 13 in]
          }
          event "Load Config": Value Change {
            n63 = event-data() -> ()  [unwired: 1 in, 6 out]
            n64 = call <vilib>:"Add State(s) to Queue__jki_lib_state_machine.vi"("State(s) in (\"\")"=w155, "State(s) at Back (\"\")"="Load Configuration" ("State(s) in Front (\"\")")) -> ("States Out"=w154:string)  [unwired: 13 in]
          }
          event "Reset History": Value Change {
            n65 = event-data() -> ()  [unwired: 1 in, 6 out]
            n66 = call <vilib>:"Add State(s) to Queue__jki_lib_state_machine.vi"("State(s) in (\"\")"=w160, "State(s) at Back (\"\")"="Reset History" ("State(s) in Front (\"\")")) -> ("States Out"=w159:string)  [unwired: 13 in]
          }
          event "Set Centriod Target": Value Change {
            n67 = event-data() -> ()  [unwired: 1 in, 6 out]
            n68 = Two Button Dialog(message="Do want to update the target?") -> (T button?=w163:bool)  [unwired: 2 in]
            n69 = case shown="True" w163 {
              tunnel: w166 -> [_ w173]
              frame False {
              }
              frame True {
                n70 = Unbundle By Name(w173) -> ("Centriod X"=w172:dbl[], "Centriod Y"=w170:dbl[])
                n71 = Index Array(array=w172) -> (element=w171:dbl)  [unwired: 1 in]
                n72 = Index Array(array=w170) -> (element=w169:dbl)  [unwired: 1 in]
                n73 = property on="Target.Y::1" class="DigNum (strict)"("Val(Sgnl)"=w169) -> ()  [unwired: 2 in, 2 out]
                n74 = property on="Target.X::1" class="DigNum (strict)"("Val(Sgnl)"=w171) -> ()  [unwired: 2 in, 2 out]
              }
            }
            n75 = local write "Set Centriod Target"(FALSE ("Set Centriod Target")) -> ()
          }
          event "calibrate": Value Change {
            n76 = event-data() -> ()  [unwired: 1 in, 6 out]
            n77 = call "Calibration Details"() -> ("Number of Steps"=w175:dbl, "OK"=w174:bool)  [unwired: 17 in, 1 out]
            n78 = local write "calibrate"(FALSE ("Set Centriod Target")) -> ()
            n79 = case shown="True" w174 {
              tunnel: w177 -> [w181 w188]
              tunnel: [w181 w187] -> w176
              tunnel: w175 -> [_ w183]
              frame False {
              }
              frame True {
                n80 = To Word Integer(number=w183) -> (16bit integer=w182:i16)
                n81 = Number To Decimal String(number=w182) -> (decimal integer string=w184:string)  [unwired: 1 in]
                n82 = call <vilib>:"Build State String with Arguments__jki_lib_state_machine.vi"("Arguments (\"\")"=w184, "State"="Calibrate" ("State(s) at Back (\"\")")) -> ("State with Arguments"=w185:string)  [unwired: 4 in]
                n83 = call <vilib>:"Add State(s) to Queue__jki_lib_state_machine.vi"("State(s) in (\"\")"=w188, "State(s) at Back (\"\")"=w185) -> ("States Out"=w187:string)  [unwired: 13 in]
              }
            }
          }
          event "stop": Value Change {
            # "Exit Button Value Change (pressed) Event\n(this executes Macro: Exit to terminate the VI)"
            n84 = event-data() -> ()  [unwired: 1 in, 6 out]
            n85 = call <vilib>:"Add State(s) to Queue__jki_lib_state_machine.vi"("State(s) in Front (\"\")"="Macro: Exit", "State(s) in (\"\")"=w193) -> ("States Out"=w192:string)  [unwired: 13 in]
          }
          event Panel Close? {
            # "Discard the event because we'll close the front panel ourselves in Macro: Exit"
            # "Close Panel button (pressed) Event\n(this executes Macro: Exit to terminate the VI)"
            n86 = event-data() -> ()  [unwired: 1 in, 1 out]
            n87 = call <vilib>:"Add State(s) to Queue__jki_lib_state_machine.vi"("State(s) in Front (\"\")"="Macro: Exit", "State(s) in (\"\")"=w199) -> ("States Out"=w198:string)  [unwired: 13 in]
            n88 = event-data("Discard?"=TRUE) -> ()  [unwired: 1 in, 1 out]
          }
        }
      }
      frame "---------- Core ----------" {
        # "Do not put any code in this frame.\n(it is a separator no-op)"
        n89 = call <vilib>:"Add State(s) to Queue__jki_lib_state_machine.vi"("State(s) in (\"\")"=w203) -> ("States Out"=w202:string)  [unwired: 14 in]
      }
      frame Default {
        w213 = 42 items=["No error", "Argument error", "Memory is full", "Out of zone", "End of file", "File already open", "Generic file I/O error", "File not found", "File permission error", "Disk is full", "Duplicate path", "Too many files open", "System feature not enabled", "Resource file not found", "Cannot add resource", "Resource not found", "Image not found", "Image memory error", "Pen does not exist", "Config type invalid", "Config token not found", "Config parse error", "Config memory error", "Bad external code format", "Bad external code offset", "External code not present", "Null window", "Destroy window error", "Null menu", "Print aborted", "Bad print record", "Print driver error", "Windows error during printing", "Memory error during printing", "Print dialog error", "Generic print error", "Invalid device refnum", "Device not found", "Device parameter error", "Device unit error", "Cannot open device", "Device call aborted", "Generic error", "Cancelled by user", "Object ID too low", "Object ID too high", "Object not in heap", "Unknown heap", "Unknown object (invalid DefProc)", "Unknown object (DefProc not in table)", "Message out of range", "Invalid (null) method", "Unknown message", "Manager call not supported", "Bad address", "Network operation in progress", "Network operation timed out", "Connection is busy", "Network attribute not supported", "Network error", "Address in use", "System out of memory", "Connection aborted", "Connection refused", "Not connected", "Already connected", "Connection closed", "Initialization error (interapplication manager)", "Bad occurrence", "Wait on unbound occurrence handler", "Occurrence queue overflow", "Datalog type conflict", "Unused", "Unrecognized type (interapplication manager)", "Memory corrupt", "Failed to make temporary DLL", "Old CIN version", "Drag socket not found", "Failed to load drop-object", "Failed to register OLE object", "Failed to release OLE object", "Format specifier type mismatch", "Unknown format specifier", "Too few format specifiers", "Too many format specifiers", "Scan failed", "Newer CIN version", "Error converting to variant", "Runtime menu error", "Password tampered", "Variant attribute not found", "Incompatible variant data type", "Event data is not available", "Event Store is not present", "Occurrence is not found", "Event Queue is not created", "Event info is not available", "Refnum passed is NULL", "Error retrieving Class GUID", "Error retrieving CoClass GUID", "Error retrieving TypeLib GUID.", "Bad built application magic bytes.", "Specific driver is different from the specific driver associated with the Logical Name.", "There is no session opened to the class driver.", "Max Error", "MAX - Error with config objects", "MAX - Error loading configuration", "MAX - Group not supported"]
        # "Current State"
        # "Do not delete, rename, or modify this frame.\n(this is used to capture unhandled states and typos)"
        # "Handle mistyped state name (developer tool)"
        n90 = Format Into String(format string="Software Exception: Unhandled State \"%s\"." ("message"), error in=w209, w204) -> (resulting string=w212:string, error out=w211:errorcluster)  [unwired: 1 in]
        n91 = call <vilib>:"Error Cluster From Error Code.vi"("show call chain? (False)"=TRUE, "error in (no error)"=w211, "error message (\"\")"=w212, "error code (0)"=w213) -> ("error out"=w210:errorcluster)  [unwired: 5 in]
        n92 = call <vilib>:"Add State(s) to Queue__jki_lib_state_machine.vi"("State(s) in (\"\")"=w208) -> ("States Out"=w207:string)  [unwired: 14 in]
      }
      frame "Initialize Core Data" {
        # "Do not delete, rename, or modify this frame.\n(this is used to determine panel behavior on exit)"
        # "originally closed?"
        # "exe?"
        # "If panel starts closed or is an EXE, then close it when we exit"
        n93 = property class="VI"() -> ("Front Panel.Open"=w222:bool)  [unwired: 2 in, 2 out]
        n94 = property class="App"() -> ("App.Kind"=w221:T15)  [unwired: 2 in, 2 out]
        n95 = control-ref of="Current VI Reference"() -> (w215:refnum<vi>)
        n96 = Not(x=w222) -> (.not. x?=w219:bool)
        n97 = Equal?(x=w221, y=T15."Run Time System" ("Application:Kind")) -> (x = y?=w218:bool)
        n98 = Or(x=w219, y=w218) -> (x .or. y?=w216:bool)
        n99 = Bundle By Name(cluster=w217, "Core.Current VI Reference"=w215, "Core.Close Panel on Exit?"=w216) -> (w224:T19)
        n100 = call <vilib>:"Add State(s) to Queue__jki_lib_state_machine.vi"("State(s) in (\"\")"=w226) -> ("States Out"=w225:string)  [unwired: 14 in]
      }
      frame "Error Handler" {
        # "Unhandled Error -- Display it"
        # "Handle any errors here.\nYou can also output any states to clean-up after errors occur"
        # "Clear error"
        n101 = call <vilib>:"General Error Handler.vi"("error in (no error)"=w228) -> ()  [unwired: 10 in, 5 out]
        n102 = call <vilib>:"Add State(s) to Queue__jki_lib_state_machine.vi"("State(s) in Front (\"\")"="/* Post Error States", "State(s) in (\"\")"=w232) -> ("States Out"=w231:string)  [unwired: 13 in]
      }
      frame "Exit" {
        # "Do not put any code in this frame.\n(No errors that occur here will be handled.)"
        n103 = call <vilib>:"Add State(s) to Queue__jki_lib_state_machine.vi"("State(s) in (\"\")"=w237) -> ("States Out"=w236:string)  [unwired: 14 in]
      }
      frame "---------- Data ----------" {
        # "Do not put any code in this frame.\n(It is a separator no-op. You can make a copy of this frame to create a new Data frame)"
        n104 = call <vilib>:"Add State(s) to Queue__jki_lib_state_machine.vi"("State(s) in (\"\")"=w241) -> ("States Out"=w240:string)  [unwired: 14 in]
      }
      frame "Data: Initialize" {
        w247 = T18 {"Slope Axis 1"=0.0, "Axis Inverted"=FALSE, "Slope Axis 2"=0.0, "Axis 1 revered"=FALSE, "Axis 2 revered"=FALSE}  # Motor Calibration
        w248 = FALSE  # set centriod target
        w249 = T1 {"Stat Centriod X"=[], "Stat Centriod Y"=[], "TRA Position X"=[], "TRA PositionY"=[], "Time"=[]}  # Stats
        w251 = FALSE  # moving
        w243 = T5 {"Tolerance [%]"=0.0, "Stepsize"=0.0, "Invert Axis"=FALSE, "Invert Direction X"=FALSE, "Invert Direction Y"=FALSE, "enable feedback"=FALSE, "Set Centriod Target"=FALSE, "my active motor"=""}  # move
        w252 = cluster{"X offset":dbl, "Y offset":dbl} {"X offset"=0.0, "Y offset"=0.0}  # offsets
        w253 = FALSE  # beam detected
        w250 = T3 {"Filter"=1, "Filter Para"={"X Size"=5, "Y Size"=5, "% Tolerance"=1}, "detection method"=4, "smal para"=[{"Measurement Parameter"=35, "Range Lower Value"=0.0, "Range Upper Value"=500.0, "Range"=TRUE, "Measurement Type"=FALSE}], "Remove small Objects"=TRUE, "Restrict to round Objects"=FALSE}  # beam detection para
        w255 = dbl[] []  # Mean Centriod Y
        w256 = dbl[] []  # Mean Centriod X
        w257 = T8 [{"Area"=1104.0, "Number of Holes"=0.0, "Bounding Rect"={"Left"=378.0, "Top"=230.0, "Right"=422.0, "Bottom"=264.0}, "Center of Mass"={"X"=399.60235507246375, "Y"=246.169384057971}, "Orientation"=6.346766143267859, "Dimensions"={"Width"=44.0, "Height"=34.0}}]  # PArticle Report
        w258 = T9 []  # Best Rectangle
        w259 = dbl[] []  # Centriod Y
        w260 = dbl[] []  # Centriod X
        w261 = T21 {"Current VI Reference"=refnum, "Close Panel on Exit?"=FALSE}  # Core
        # "Initialize the shift-register data, here.\n(data names are defined by what you wire into the bundle function)"
        n105 = local read "ActiveMotor"() -> (w245:u16)
        n106 = local write "beam detection para"(w250) -> ()
        n107 = property on="ActiveMotor" class="Ring (strict)"() -> ("Strings []"=w246:string[])  [unwired: 2 in, 2 out]
        n108 = Bundle("Core"=w261, "beam detection para"=w250, "Centriod X"=w260, "Centriod Y"=w259, "Best Rectangle"=w258, "PArticle Report"=w257, "Mean Centriod X"=w256, "Mean Centriod Y"=w255, "Time"="Time", "beam detected"=w253, "offsets"=w252, "move"=w243, "moving"=w251, "Stats"=w249, "set centriod target"=w248, "Motor Calibration"=w247) -> (w263:T19)  [unwired: 1 in]
        n109 = Index Array(array=w246, index=w245) -> (element=w244:string)
        n110 = Bundle By Name(cluster=w243, "my active motor"=w244) -> (w242:T5)
        n111 = property on="ActiveMotorName::2" class="Str"("Val(Sgnl)"=w244) -> ()  [unwired: 2 in, 2 out]
        n112 = call <vilib>:"Add State(s) to Queue__jki_lib_state_machine.vi"("State(s) in (\"\")"=w265) -> ("States Out"=w264:string)  [unwired: 14 in]
        n113 = property on="Move Properties" class="Clust (strict)"("Value"=w242) -> ()  [unwired: 2 in, 2 out]
      }
      frame "Data: Cleanup" {
        # "Cleanup any data and references, here.\n(this is called automatically, by the Macro: Exit)"
        n114 = Unbundle By Name(w267) -> ("Core.Current VI Reference"=w266:refnum<vi>)
        n115 = Close Reference(reference=w266, error in (no error)=w269) -> (error out=w268:errorcluster)
        n116 = call <vilib>:"Add State(s) to Queue__jki_lib_state_machine.vi"("State(s) in (\"\")"=w271) -> ("States Out"=w270:string)  [unwired: 14 in]
      }
      frame "---------- UI ----------" {
        # "Do not put any code in this frame.\n(It is a separator no-op. You can make a copy of this frame to create a new UI frame)"
        n117 = call <vilib>:"Add State(s) to Queue__jki_lib_state_machine.vi"("State(s) in (\"\")"=w275) -> ("States Out"=w274:string)  [unwired: 14 in]
      }
      frame "UI: Initialize" {
        # "Initialize the User Interface, here.\n(this is called automatically, by the Macro: Init)"
        n118 = call <vilib>:"Add State(s) to Queue__jki_lib_state_machine.vi"("State(s) in (\"\")"=w279) -> ("States Out"=w278:string)  [unwired: 14 in]
      }
      frame "UI: Cursor Set" {
        # "Argument"
        # "Set and Unset Cursor Busy.\n(Usage: \"UI: Cursor Set >> Busy|Idle\")"
        n119 = case shown="\"Idle\", Default" w280 {
          tunnel: w282 -> [w287 w289]
          tunnel: [w286 w288] -> w281
          frame "Idle", Default {
            n120 = call <vilib>:"Unset Busy.vi"("error in (no error)"=w287) -> ("error out"=w286:errorcluster)  [unwired: 10 in]
          }
          frame "Busy" {
            n121 = call <vilib>:"Set Busy.vi"("error in (no error)"=w289) -> ("error out"=w288:errorcluster)  [unwired: 9 in, 1 out]
          }
        }
        n122 = call <vilib>:"Add State(s) to Queue__jki_lib_state_machine.vi"("State(s) in (\"\")"=w285) -> ("States Out"=w284:string)  [unwired: 14 in]
      }
      frame "UI: Front Panel State" {
        # "Argument"
        # "Set Front Panel Open or Closed\n(Usage: \"UI: Front Panel State >> Open|Close\")"
        n123 = Unbundle By Name(w292) -> ("Core.Current VI Reference"=w291:refnum<vi>)
        n124 = case shown="\"Close\"" w290 {
          tunnel: w294 -> [w300 w313]
          tunnel: [w302 w314] -> w293
          tunnel: w291 -> [w301 w311]
          frame "Open", Default {
            n125 = property class="VI"(reference=w301, error in=w300) -> (reference out=w298:refnum<vi>, error out=w299:errorcluster, "Front Panel.Open"=w297:bool)
            n126 = case shown="False" w297 {
              tunnel: [w305 w308] -> w302
              tunnel: w299 -> [w304 w308]
              tunnel: w298 -> [w303 _]
              frame False {
                n127 = invoke class="VI" method="FP.Open"(reference=w303, error in=w304, "Activate"=TRUE, "State"=T16."Standard") -> (error out=w305:errorcluster)  [unwired: 1 in, 4 out]
              }
              frame True {
              }
            }
          }
          frame "Close" {
            n128 = property class="VI"(reference=w311, error in=w313) -> (reference out=w310:refnum<vi>, error out=w312:errorcluster, "Front Panel.Open"=w309:bool)
            n129 = case shown="True" w309 {
              tunnel: [w315 w318] -> w314
              tunnel: w312 -> [w315 w317]
              tunnel: w310 -> [_ w316]
              frame False {
              }
              frame True {
                n130 = invoke class="VI" method="FP.Close"(reference=w316, error in=w317) -> (error out=w318:errorcluster)  [unwired: 1 in, 2 out]
              }
            }
          }
        }
        n131 = call <vilib>:"Add State(s) to Queue__jki_lib_state_machine.vi"("State(s) in (\"\")"=w296) -> ("States Out"=w295:string)  [unwired: 14 in]
      }
      frame "---------- Macro ----------" {
        # "Do not put any code in this frame.\n(It is a separator no-op. You can make a copy of this frame to create a new Macro frame)"
        n132 = call <vilib>:"Add State(s) to Queue__jki_lib_state_machine.vi"("State(s) in (\"\")"=w322) -> ("States Out"=w321:string)  [unwired: 14 in]
      }
      frame "Macro: Initialize" {
        w323 = "Data: Initialize\nInitialize Core Data\nUI: Initialize\nUI: Front Panel State >> Open"  # Data: Initialize Initialize Core Data UI: Initialize UI: Front Panel State >> Open
        # "Initialization Macro\n(This is called once, when the VI starts)"
        n133 = call <vilib>:"Add State(s) to Queue__jki_lib_state_machine.vi"("State(s) in Front (\"\")"=w323, "State(s) in (\"\")"=w327) -> ("States Out"=w326:string)  [unwired: 13 in]
      }
      frame "Macro: Exit" {
        # "Exit Macro\n(This is called once, when the VI exits)"
        n134 = Unbundle By Name(w334) -> ("Core.Close Panel on Exit?"=w332:bool)
        n135 = Select(t="UI: Front Panel State >> Close", s=w332, f="") -> (s? t:f=w329:string)
        n136 = call <vilib>:"Add State(s) to Queue__jki_lib_state_machine.vi"("State(s) in (\"\")"=w329, "State(s) at Back (\"\")"="Data: Cleanup\nExit") -> ("States Out"=w333:string)  [unwired: 13 in]
        n137 = call <vilib>:"Add State(s) to Queue__jki_lib_state_machine.vi"("State(s) in Front (\"\")"=w333, "State(s) in (\"\")"=w337) -> ("States Out"=w336:string)  [unwired: 13 in]
      }
      frame "-------------Properties---------" {
        # "Template Separator\n(You can make a copy of, or modify, this frame)"
        n138 = call <vilib>:"Add State(s) to Queue__jki_lib_state_machine.vi"("State(s) in (\"\")"=w341) -> ("States Out"=w340:string)  [unwired: 14 in]
      }
      frame "Beam Detection" {
        # "Your code here.\n(You can make a copy of, or modify, this frame)"
        n139 = Bundle By Name(cluster=w343, "beam detection para"="beam detection para") -> (w342:T19)
        n140 = call <vilib>:"Add State(s) to Queue__jki_lib_state_machine.vi"("State(s) in (\"\")"=w347) -> ("States Out"=w346:string)  [unwired: 14 in]
      }
      frame "Move Properties" {
        n141 = Bundle By Name(cluster=w350, "move"="Move Properties") -> (w349:T19)
        n142 = Unbundle By Name(w349) -> ("move.Stepsize"=w348:dbl)
        n143 = property on="RelativeSettings.Axis 1.StepSize::2" class="DigNum (strict)"("Val(Sgnl)"=w348) -> ()  [unwired: 2 in, 2 out]
        n144 = property on="RelativeSettings.Axis 2.StepSize::2" class="DigNum (strict)"("Val(Sgnl)"=w348) -> ()  [unwired: 2 in, 2 out]
        n145 = call <vilib>:"Add State(s) to Queue__jki_lib_state_machine.vi"("State(s) in (\"\")"=w354) -> ("States Out"=w353:string)  [unwired: 14 in]
      }
      frame "Save Configuration" {
        n146 = Bundle By Name(cluster=w358, "move.enable feedback"=FALSE) -> (w356:T19)
        n147 = local read "GUIdevice 1"() -> (w361:string)
        n148 = local read "ActiveMotor"() -> (w359:u16)
        n149 = local read "GUIdevice 2"() -> (w360:string)
        n150 = local read "stats path"() -> (w355:path)
        n151 = Unbundle By Name(w356) -> ("beam detection para"=w370:T3, "move"=w369:T5)
        n152 = local read "img to avg"() -> (w371:i32)
        n153 = Bundle("img to avg"=w371, "beam detection para"=w370, "move"=w369, "GUIdevice 1"=w361, "GUIdevice 2"=w360, "ActiveMotor"=w359, "stats path"=w355) -> (w368:T6)  [unwired: 1 in]
        n154 = Open/Create/Replace File(error in=w364, operation (0:open)=T17."replace or create with confirmation") -> (refnum out=w372:refnum<file>, error out=w367:errorcluster)  [unwired: 4 in, 1 out]
        n155 = Write to Binary File(file (use dialog)=w372, data=w368, error in=w367) -> (refnum out=w365:refnum<file>, error out=w366:errorcluster)  [unwired: 3 in, 1 out]
        n156 = Close File(refnum=w365, error in=w366) -> (error out=w363:errorcluster)  [unwired: 1 out]
        n157 = local write "Save Config"(FALSE ("Save Button")) -> ()
        n158 = call <vilib>:"Add State(s) to Queue__jki_lib_state_machine.vi"("State(s) in (\"\")"=w375) -> ("States Out"=w374:string)  [unwired: 14 in]
      }
      frame "Save Stats" {
        n159 = local read "Save Stats"() -> (w376:bool)
        n160 = Unbundle By Name(w381) -> ("Stats"=w377:T1)
        n161 = case shown="True" w376 {
          tunnel: w380 -> [w384 w388]
          tunnel: [w384 w387] -> w379
          tunnel: w377 -> [_ w386]
          frame False {
          }
          frame True {
            n162 = Open/Create/Replace File(file path (use dialog)="stats path", error in=w388, operation (0:open)=T17."replace or create") -> (refnum out=w392:refnum<file>, error out=w391:errorcluster)  [unwired: 3 in, 1 out]
            n163 = Write to Binary File(file (use dialog)=w392, data=w386, error in=w391) -> (refnum out=w389:refnum<file>, error out=w390:errorcluster)  [unwired: 3 in, 1 out]
            n164 = Close File(refnum=w389, error in=w390) -> (error out=w387:errorcluster)  [unwired: 1 out]
          }
        }
        n165 = call <vilib>:"Add State(s) to Queue__jki_lib_state_machine.vi"("State(s) in (\"\")"=w383) -> ("States Out"=w382:string)  [unwired: 14 in]
        n166 = local write "Save Stats"(FALSE ("Save Button")) -> ()
      }
      frame "Save Centriod" {
        n167 = local read "Save Stats"() -> (w394:bool)
        n168 = Unbundle By Name(w402) -> ("Time"=w398:timestamp[], "Mean Centriod X"=w397:dbl[], "Mean Centriod Y"=w396:dbl[])
        n169 = Bundle("Time"=w398, "Mean Centriod X"=w397, "Mean Centriod Y"=w396) -> (w395:T2)  [unwired: 1 in]
        n170 = case shown="True" w394 {
          tunnel: w401 -> [w405 w414]
          tunnel: [w405 w413] -> w400
          tunnel: w395 -> [_ w406]
          frame False {
          }
          frame True {
            n171 = local read "stats path"() -> (w412:path)
            n172 = Strip Path(path=w412) -> (stripped path=w408:path, name=w411:string)
            n173 = Concatenate Strings("Centriod_" ("string"), w411) -> (w409:string)
            n174 = Build Path(base path=w408, name or relative path=w409) -> (appended path=w407:path)
            n175 = Open/Create/Replace File(file path (use dialog)=w407, error in=w414, operation (0:open)=T17."replace or create") -> (refnum out=w418:refnum<file>, error out=w417:errorcluster)  [unwired: 3 in, 1 out]
            n176 = Write to Binary File(file (use dialog)=w418, data=w406, error in=w417) -> (refnum out=w415:refnum<file>, error out=w416:errorcluster)  [unwired: 3 in, 1 out]
            n177 = Close File(refnum=w415, error in=w416) -> (error out=w413:errorcluster)  [unwired: 1 out]
          }
        }
        n178 = call <vilib>:"Add State(s) to Queue__jki_lib_state_machine.vi"("State(s) in (\"\")"=w404) -> ("States Out"=w403:string)  [unwired: 14 in]
        n179 = local write "Save Stats"(FALSE ("Save Button")) -> ()
      }
      frame "Load Configuration" {
        # "Your code here.\n(You can make a copy of, or modify, this frame)"
        n180 = Open/Create/Replace File(error in=w430, operation (0:open)=T17."open") -> (refnum out=w437:refnum<file>, error out=w436:errorcluster)  [unwired: 4 in, 1 out]
        n181 = Read from Binary File(5:"output cluster", 8:w436, 11:w437) -> (0:w435:errorcluster, 2:w433:T6, 3:w434:refnum<file>)  [unwired: 3 in, 1 out]
        n182 = Close File(refnum=w434, error in=w435) -> (error out=w429:errorcluster)  [unwired: 1 out]
        n183 = Unbundle By Name(w433) -> ("img to avg"=w422:i32, "beam detection para"=w428:T3, "move"=w427:T5, "GUIdevice 1"=w425:string, "GUIdevice 2"=w424:string, "ActiveMotor"=w421:u16, "stats path"=w420:path)
        n184 = local write "img to avg"(w422) -> ()
        n185 = property on="GUIdevice 2" class="Str"("Val(Sgnl)"=w424) -> ()  [unwired: 2 in, 2 out]
        n186 = local write "ActiveMotor"(w421) -> ()
        n187 = local write "stats path"(w420) -> ()
        n188 = property on="GUIdevice 1" class="Str"("Val(Sgnl)"=w425) -> ()  [unwired: 2 in, 2 out]
        n189 = call <vilib>:"Add State(s) to Queue__jki_lib_state_machine.vi"("State(s) in (\"\")"=w440) -> ("States Out"=w439:string)  [unwired: 14 in]
        n190 = Bundle By Name(cluster=w432, "beam detection para"=w428, "move"=w427) -> (w431:T19)
        n191 = local write "Load Config"(FALSE ("Load Button")) -> ()
        n192 = local write "beam detection para"(w428) -> ()
        n193 = local write "Move Properties"(w427) -> ()
      }
      frame "Reset History" {
        w445 = dbl[] [] ("Mean Centriod X")
        # "Your code here.\n(You can make a copy of, or modify, this frame)"
        n194 = local write "Reset History"(FALSE ("Reset History")) -> ()
        n195 = call <vilib>:"Add State(s) to Queue__jki_lib_state_machine.vi"("State(s) in (\"\")"=w448) -> ("States Out"=w447:string)  [unwired: 14 in]
        n196 = Bundle By Name(cluster=w444, "Mean Centriod X"=w445, "Mean Centriod Y"=w445, "Stats"=T1 {"Stat Centriod X"=[], "Stat Centriod Y"=[], "TRA Position X"=[], "TRA PositionY"=[], "Time"=[]}) -> (w443:T19)
      }
      frame "---------- centriod analysis----------" {
        # "Template Separator\n(You can make a copy of, or modify, this frame)"
        n197 = call <vilib>:"Add State(s) to Queue__jki_lib_state_machine.vi"("State(s) in (\"\")"=w452) -> ("States Out"=w451:string)  [unwired: 14 in]
      }
      frame "detected" {
        w458 = 101 ("y")
        w483 = dbl[] [] ("Array")
        n198 = Unbundle By Name(w468) -> ("Time"=w476:timestamp[], "Centriod X"=w471:dbl[], "Mean Centriod X"=w475:dbl[], "Centriod Y"=w470:dbl[], "Mean Centriod Y"=w474:dbl[], "Best Rectangle"=→"Best Rectangle":T9)
        n199 = local read "Target.X::1"() -> (w473:dbl)
        n200 = local read "Target.Y::1"() -> (w472:dbl)
        n201 = call <vilib>:"Std Deviation and Variance.vi"("X"=w471) -> ("mean"=w477:dbl)  [unwired: 1 in, 2 out]
        "mean X" <- w477
        n202 = call <vilib>:"Std Deviation and Variance.vi"("X"=w470) -> ("mean"=w478:dbl)  [unwired: 1 in, 2 out]
        "mean Y" <- w478
        n203 = Subtract(x=w473, y=w477) -> (x-y=w466:dbl)
        "X offset" <- w466
        n204 = Subtract(x=w472, y=w478) -> (x-y=w465:dbl)
        "Y offset" <- w465
        n205 = Get Date/Time In Seconds() -> (seconds since 1Jan1904=w479:timestamp)
        n206 = Build Array (concatenate)(w475, w466) -> (w455:dbl[])
        n207 = Build Array (concatenate)(w474, w465) -> (w456:dbl[])
        n208 = Build Array (concatenate)(w476, w479) -> (w469:timestamp[])
        n209 = Bundle(w466, w465) -> (w464:cluster{dbl, dbl})  [unwired: 1 in]
        n210 = Array Size(array=w455) -> (size(s)=w460:i32)
        n211 = call <vilib>:"Add State(s) to Queue__jki_lib_state_machine.vi"("State(s) in (\"\")"=w485, "State(s) at Back (\"\")"="check move") -> ("States Out"=w454:string)  [unwired: 13 in]
        n212 = Decrement(x=w458) -> (x-1=w457:i32)
        n213 = Quotient & Remainder(x=w460, y=w458) -> (x-y*floor(x/y)=w459:i32)  [unwired: 1 out]
        n214 = Bundle(w469, w455) -> (w480:cluster{timestamp[], dbl[]})  [unwired: 1 in]
        n215 = Bundle(w469, w456) -> (w481:cluster{timestamp[], dbl[]})  [unwired: 1 in]
        n216 = Equal?(x=w459, y=w457) -> (x = y?=w461:bool)
        n217 = Build Array(w480, w481) -> (→"XY Graph":cluster{timestamp[], dbl[]}[])
        n218 = case shown="True" w461 {
          tunnel: [w486 w488] -> w453
          tunnel: w454 -> [w486 w487]
          frame False {
          }
          frame True {
            n219 = call <vilib>:"Add State(s) to Queue__jki_lib_state_machine.vi"("State(s) in Front (\"\")"=w487, "State(s) at Back (\"\")"="Save Centriod" ("State(s) at Back (\"\")")) -> ("States Out"=w488:string)  [unwired: 13 in]
          }
        }
        n220 = Bundle By Name(cluster=w468, "Time"=w469, "Mean Centriod X"=w455, "Mean Centriod Y"=w456, "Centriod X"=w483, "Centriod Y"=w483, "offsets"=w464) -> (w467:T19)
      }
      frame "check move" {
        n221 = Unbundle By Name(w497) -> ("Best Rectangle"=w515:T9, "offsets.X offset"=w514:dbl, "offsets.Y offset"=w513:dbl)
        n222 = Absolute Value(x=w514) -> (abs(x)=w510:dbl)
        n223 = Absolute Value(x=w513) -> (abs(x)=w507:dbl)
        n224 = Unbundle By Name(w497) -> ("move.Tolerance [%]"=w512:dbl)
        n225 = call "Beam Size.vi"("Best Rectangle"=w515) -> ("Y Size"=w493:dbl, "X Size"=w494:dbl)  [unwired: 9 in]
        "X Size" <- w494
        "Y Size" <- w493
        n226 = Divide(x=w512, y=100.0) -> (x/y=w508:dbl)
        n227 = Max & Min(x=w494, y=w493) -> (max(x,y)=w492:dbl)  [unwired: 1 out]
        n228 = Multiply(x=w508, y=w494) -> (x*y=w509:dbl)
        n229 = Multiply(x=w508, y=w493) -> (x*y=w506:dbl)
        n230 = Divide(x=w492, y=2.0) -> (x/y=w490:dbl)
        n231 = local write "size"(w490) -> ()
        n232 = Greater Or Equal?(x=w510, y=w509) -> (x >= y?=w500:bool)
        n233 = Greater Or Equal?(x=w507, y=w506) -> (x >= y?=w499:bool)
        n234 = Unbundle By Name(w497) -> ("move.enable feedback"=w496:bool)
        n235 = case shown="True" w499 {
          tunnel: w495 -> [w521 w524]
          tunnel: [w521 w522] -> w505
          frame False {
          }
          frame True {
            n236 = call <vilib>:"Add State(s) to Queue__jki_lib_state_machine.vi"("State(s) in (\"\")"=w524, "State(s) at Back (\"\")"="Move Y" ("State(s) at Back (\"\")")) -> ("States Out"=w522:string)  [unwired: 13 in]
          }
        }
        n237 = case shown="True" w500 {
          tunnel: w495 -> [w525 w528]
          tunnel: [w525 w526] -> w504
          frame False {
          }
          frame True {
            n238 = call <vilib>:"Add State(s) to Queue__jki_lib_state_machine.vi"("State(s) in (\"\")"=w528, "State(s) at Back (\"\")"="Move X" ("State(s) at Back (\"\")")) -> ("States Out"=w526:string)  [unwired: 13 in]
          }
        }
        n239 = Or(x=w500, y=w499) -> (x .or. y?=w498:bool)
        n240 = local write "move required"(w498) -> ()
        n241 = Bundle By Name(cluster=w497, "Best Rectangle"=T9 []) -> (w501:T19)
        n242 = case shown="True" w496 {
          tunnel: w505 -> [_ w520]
          tunnel: w504 -> [_ w519]
          tunnel: [w517 w518] -> w503
          tunnel: w495 -> [w517 _]
          frame False {
          }
          frame True {
            n243 = call <vilib>:"Add State(s) to Queue__jki_lib_state_machine.vi"("State(s) in (\"\")"=w519, "State(s) at Back (\"\")"=w520) -> ("States Out"=w518:string)  [unwired: 13 in]
          }
        }
      }
      frame "-----------Motor Move---------" {
        # "Your code here.\n(You can make a copy of, or modify, this frame)"
        n244 = call <vilib>:"Add State(s) to Queue__jki_lib_state_machine.vi"("State(s) in (\"\")"=w532) -> ("States Out"=w531:string)  [unwired: 14 in]
      }
      frame "Move X" {
        w552 = TRUE ("moving")
        n245 = Unbundle By Name(w548) -> ("RelativeMove.Axis 1.CW::2"=w547:refnum<vi>, "RelativeMove.Axis 1.CCW::2"=w546:refnum<vi>, "RelativeMove.Axis 2.CW::2"=w545:refnum<vi>, "RelativeMove.Axis 2.CCW::2"=w544:refnum<vi>)
        n246 = Unbundle By Name(w543) -> ("move.Invert Direction X"=w549:bool, "move.Invert Axis"=w550:bool, "offsets.X offset"=w551:dbl)
        n247 = Greater Than 0?(x=w551) -> (x > 0?=w541:bool)
        n248 = Unbundle By Name(w543) -> ("move.my active motor"=w542:string)
        n249 = stacked-sequence {
          tunnel: w541 -> [_ w564]
          tunnel: w550 -> [_ w563]
          tunnel: w549 -> [_ w562]
          tunnel: w547 -> [_ w561]
          tunnel: w546 -> [_ w560]
          tunnel: w545 -> [_ w559]
          tunnel: w544 -> [_ w558]
          tunnel: w542 -> [w557 _]
          frame #0 {
            n250 = property on="ActiveMotorName::2" class="Str"("Val(Sgnl)"=w557) -> ()  [unwired: 2 in, 2 out]
          }
          frame #1 {
            n251 = case shown="True" w564 {
              tunnel: w563 -> [w570 w590]
              tunnel: w562 -> [w569 w589]
              tunnel: w561 -> [w568 w587]
              tunnel: w560 -> [w567 w588]
              tunnel: w559 -> [w566 w586]
              tunnel: w558 -> [w565 w585]
              frame True {
                n252 = case shown="False" w570 {
                  tunnel: w569 -> [w573 w580]
                  tunnel: w568 -> [w572 _]
                  tunnel: w567 -> [w571 _]
                  tunnel: w566 -> [_ w579]
                  tunnel: w565 -> [_ w578]
                  frame False {
                    n253 = case shown="False" w573 {
                      tunnel: w572 -> [w575 _]
                      tunnel: w571 -> [_ w576]
                      frame False {
                        n254 = property class="Bool (strict)"(reference=w575, "Val(Sgnl)"=TRUE ("Value (Signaling)")) -> ()  [unwired: 1 in, 2 out]
                      }
                      frame True {
                        n255 = property class="Bool (strict)"(reference=w576, "Val(Sgnl)"=TRUE ("Value (Signaling)")) -> ()  [unwired: 1 in, 2 out]
                      }
                    }
                  }
                  frame True {
                    n256 = case shown="False" w580 {
                      tunnel: w579 -> [w581 _]
                      tunnel: w578 -> [_ w583]
                      frame False {
                        n257 = property class="Bool (strict)"(reference=w581, "Val(Sgnl)"=TRUE ("Value (Signaling)")) -> ()  [unwired: 1 in, 2 out]
                      }
                      frame True {
                        n258 = property class="Bool (strict)"(reference=w583, "Val(Sgnl)"=TRUE ("Value (Signaling)")) -> ()  [unwired: 1 in, 2 out]
                      }
                    }
                  }
                }
              }
              frame False {
                n259 = case shown="True" w590 {
                  tunnel: w589 -> [w593 w600]
                  tunnel: w588 -> [w592 _]
                  tunnel: w587 -> [w591 _]
                  tunnel: w586 -> [_ w599]
                  tunnel: w585 -> [_ w598]
                  frame False {
                    n260 = case shown="True" w593 {
                      tunnel: w592 -> [w594 _]
                      tunnel: w591 -> [_ w596]
                      frame False {
                        n261 = property class="Bool (strict)"(reference=w594, "Val(Sgnl)"=TRUE ("Value (Signaling)")) -> ()  [unwired: 1 in, 2 out]
                      }
                      frame True {
                        n262 = property class="Bool (strict)"(reference=w596, "Val(Sgnl)"=TRUE ("Value (Signaling)")) -> ()  [unwired: 1 in, 2 out]
                      }
                    }
                  }
                  frame True {
                    n263 = case shown="True" w600 {
                      tunnel: w599 -> [w601 _]
                      tunnel: w598 -> [_ w603]
                      frame False {
                        n264 = property class="Bool (strict)"(reference=w601, "Val(Sgnl)"=TRUE ("Value (Signaling)")) -> ()  [unwired: 1 in, 2 out]
                      }
                      frame True {
                        n265 = property class="Bool (strict)"(reference=w603, "Val(Sgnl)"=TRUE ("Value (Signaling)")) -> ()  [unwired: 1 in, 2 out]
                      }
                    }
                  }
                }
              }
            }
          }
        }
        n266 = Select(t="pos", s=w541, f="neg") -> (s? t:f=w538:string)
        n267 = Concatenate Strings("x" ("string"), w538) -> (w536:string)
        n268 = call <vilib>:"Build State String with Arguments__jki_lib_state_machine.vi"("Arguments (\"\")"=w536, "State"="Stats") -> ("State with Arguments"=w534:string)  [unwired: 4 in]
        n269 = call <vilib>:"Add State(s) to Queue__jki_lib_state_machine.vi"("State(s) in Front (\"\")"="Wait", "State(s) in (\"\")"=w556, "State(s) at Back (\"\")"=w534) -> ("States Out"=w555:string)  [unwired: 12 in]
        n270 = Bundle By Name(cluster=w543, "moving"=w552) -> (w553:T19)
        n271 = local write "moving"(w552) -> ()
      }
      frame "Move Y" {
        w624 = TRUE ("moving")
        n272 = Unbundle By Name(w620) -> ("RelativeMove.Axis 2.CW::2"=w619:refnum<vi>, "RelativeMove.Axis 2.CCW::2"=w618:refnum<vi>, "RelativeMove.Axis 1.CW::2"=w617:refnum<vi>, "RelativeMove.Axis 1.CCW::2"=w616:refnum<vi>)
        n273 = Unbundle By Name(w615) -> ("move.Invert Direction Y"=w621:bool, "move.Invert Axis"=w622:bool, "offsets.Y offset"=w623:dbl)
        n274 = Greater Than 0?(x=w623) -> (x > 0?=w609:bool)
        n275 = Unbundle By Name(w615) -> ("move.my active motor"=w614:string)
        n276 = stacked-sequence {
          tunnel: w609 -> [_ w636]
          tunnel: w622 -> [_ w635]
          tunnel: w621 -> [_ w634]
          tunnel: w619 -> [_ w633]
          tunnel: w618 -> [_ w632]
          tunnel: w617 -> [_ w631]
          tunnel: w616 -> [_ w630]
          tunnel: w614 -> [w629 _]
          frame #0 {
            n277 = property on="ActiveMotorName::2" class="Str"("Val(Sgnl)"=w629) -> ()  [unwired: 2 in, 2 out]
          }
          frame #1 {
            n278 = case shown="True" w636 {
              tunnel: w635 -> [w642 w662]
              tunnel: w634 -> [w641 w661]
              tunnel: w633 -> [w640 w659]
              tunnel: w632 -> [w639 w660]
              tunnel: w631 -> [w638 w658]
              tunnel: w630 -> [w637 w657]
              frame True {
                n279 = case shown="True" w642 {
                  tunnel: w641 -> [w645 w652]
                  tunnel: w640 -> [w644 _]
                  tunnel: w639 -> [w643 _]
                  tunnel: w638 -> [_ w651]
                  tunnel: w637 -> [_ w650]
                  frame False {
                    n280 = case shown="False" w645 {
                      tunnel: w644 -> [w647 _]
                      tunnel: w643 -> [_ w648]
                      frame False {
                        n281 = property class="Bool (strict)"(reference=w647, "Val(Sgnl)"=TRUE ("Value (Signaling)")) -> ()  [unwired: 1 in, 2 out]
                      }
                      frame True {
                        n282 = property class="Bool (strict)"(reference=w648, "Val(Sgnl)"=TRUE ("Value (Signaling)")) -> ()  [unwired: 1 in, 2 out]
                      }
                    }
                  }
                  frame True {
                    n283 = case shown="True" w652 {
                      tunnel: w651 -> [w653 _]
                      tunnel: w650 -> [_ w655]
                      frame False {
                        n284 = property class="Bool (strict)"(reference=w653, "Val(Sgnl)"=TRUE ("Value (Signaling)")) -> ()  [unwired: 1 in, 2 out]
                      }
                      frame True {
                        n285 = property class="Bool (strict)"(reference=w655, "Val(Sgnl)"=TRUE ("Value (Signaling)")) -> ()  [unwired: 1 in, 2 out]
                      }
                    }
                  }
                }
              }
              frame False {
                n286 = case shown="True" w662 {
                  tunnel: w661 -> [w665 w672]
                  tunnel: w660 -> [w664 _]
                  tunnel: w659 -> [w663 _]
                  tunnel: w658 -> [_ w671]
                  tunnel: w657 -> [_ w670]
                  frame False {
                    n287 = case shown="True" w665 {
                      tunnel: w664 -> [w666 _]
                      tunnel: w663 -> [_ w668]
                      frame False {
                        n288 = property class="Bool (strict)"(reference=w666, "Val(Sgnl)"=TRUE ("Value (Signaling)")) -> ()  [unwired: 1 in, 2 out]
                      }
                      frame True {
                        n289 = property class="Bool (strict)"(reference=w668, "Val(Sgnl)"=TRUE ("Value (Signaling)")) -> ()  [unwired: 1 in, 2 out]
                      }
                    }
                  }
                  frame True {
                    n290 = case shown="True" w672 {
                      tunnel: w671 -> [w673 _]
                      tunnel: w670 -> [_ w675]
                      frame False {
                        n291 = property class="Bool (strict)"(reference=w673, "Val(Sgnl)"=TRUE ("Value (Signaling)")) -> ()  [unwired: 1 in, 2 out]
                      }
                      frame True {
                        n292 = property class="Bool (strict)"(reference=w675, "Val(Sgnl)"=TRUE ("Value (Signaling)")) -> ()  [unwired: 1 in, 2 out]
                      }
                    }
                  }
                }
              }
            }
          }
        }
        n293 = Select(t="pos", s=w609, f="neg") -> (s? t:f=w611:string)
        n294 = Concatenate Strings("y" ("string"), w611) -> (w607:string)
        n295 = call <vilib>:"Build State String with Arguments__jki_lib_state_machine.vi"("Arguments (\"\")"=w607, "State"="Stats") -> ("State with Arguments"=w605:string)  [unwired: 4 in]
        n296 = call <vilib>:"Add State(s) to Queue__jki_lib_state_machine.vi"("State(s) in Front (\"\")"="Wait", "State(s) in (\"\")"=w628, "State(s) at Back (\"\")"=w605) -> ("States Out"=w627:string)  [unwired: 12 in]
        n297 = Bundle By Name(cluster=w615, "moving"=w624) -> (w625:T19)
        n298 = local write "moving"(w624) -> ()
      }
      frame "Wait" {
        w686 = TRUE ("moving")
        # "Wait as long as the motor is moving"
        n299 = Unbundle By Name(w684) -> ("move.Stepsize"=w683:dbl)
        n300 = Multiply(x=w683, y=1.0) -> (x*y=w681:dbl)
        n301 = Add(x=w681, y=100.0) -> (x+y=w679:dbl)
        n302 = call <userlib>:"Wait (ms)__ogtk.vi"("error in (no error)"=w678, "milliseconds to wait"=w679) -> ("error out"=w677:errorcluster)  [unwired: 8 in, 1 out]
        n303 = call <vilib>:"Add State(s) to Queue__jki_lib_state_machine.vi"("State(s) in (\"\")"=w688) -> ("States Out"=w687:string)  [unwired: 14 in]
        n304 = Bundle By Name(cluster=w684, "moving"=w686) -> (w685:T19)
        n305 = local write "moving"(w686) -> ()
      }
      frame "Stats" {
        w696 = 21 ("y")
        # "Your code here.\n(You can make a copy of, or modify, this frame)"
        n306 = Unbundle By Name(w723) -> ("move.Stepsize"=w691:dbl, "Stats.TRA Position X"=w693:dbl[], "Stats.TRA PositionY"=w692:dbl[], "Stats.Stat Centriod X"=w720:dbl[], "Mean Centriod Y"=w719:dbl[], "Stats.Time"=w716:timestamp[])
        n307 = case shown="\"xpos\", Default" w694 {
          tunnel: w693 -> [w731 w739 w748 w756]
          tunnel: w692 -> [w728 w736 w746 w754]
          tunnel: w691 -> [w732 w740 w749 w757]
          tunnel: [w730 w738 w745 w753] -> w689
          tunnel: [w727 w735 w743 w751] -> w690
          frame "xpos", Default {
            n308 = Reverse 1D Array(array=w728) -> (reversed array=w729:dbl[])
            n309 = Reverse 1D Array(array=w731) -> (reversed array=w734:dbl[])
            n310 = Index Array(array=w729) -> (element=w727:dbl)  [unwired: 1 in]
            n311 = Index Array(array=w734) -> (element=w733:dbl)  [unwired: 1 in]
            n312 = Add(x=w733, y=w732) -> (x+y=w730:dbl)
          }
          frame "xneg" {
            n313 = Reverse 1D Array(array=w736) -> (reversed array=w737:dbl[])
            n314 = Reverse 1D Array(array=w739) -> (reversed array=w742:dbl[])
            n315 = Index Array(array=w737) -> (element=w735:dbl)  [unwired: 1 in]
            n316 = Index Array(array=w742) -> (element=w741:dbl)  [unwired: 1 in]
            n317 = Subtract(x=w741, y=w740) -> (x-y=w738:dbl)
          }
          frame "yneg" {
            n318 = Reverse 1D Array(array=w746) -> (reversed array=w747:dbl[])
            n319 = Reverse 1D Array(array=w748) -> (reversed array=w750:dbl[])
            n320 = Index Array(array=w747) -> (element=w744:dbl)  [unwired: 1 in]
            n321 = Index Array(array=w750) -> (element=w745:dbl)  [unwired: 1 in]
            n322 = Subtract(x=w744, y=w749) -> (x-y=w743:dbl)
          }
          frame "ypos" {
            n323 = Reverse 1D Array(array=w754) -> (reversed array=w755:dbl[])
            n324 = Reverse 1D Array(array=w756) -> (reversed array=w758:dbl[])
            n325 = Index Array(array=w755) -> (element=w752:dbl)  [unwired: 1 in]
            n326 = Index Array(array=w758) -> (element=w753:dbl)  [unwired: 1 in]
            n327 = Add(x=w752, y=w757) -> (x+y=w751:dbl)
          }
        }
        n328 = local read "Y offset"() -> (w717:dbl)
        n329 = local read "X offset"() -> (w718:dbl)
        n330 = Get Date/Time In Seconds() -> (seconds since 1Jan1904=w715:timestamp)
        n331 = Decrement(x=w696) -> (x-1=w695:i32)
        n332 = Build Array (concatenate)(w720, w718) -> (w721:dbl[])
        n333 = Build Array (concatenate)(w719, w717) -> (w699:dbl[])
        n334 = Array Size(array=w699) -> (size(s)=w698:i32)
        n335 = Quotient & Remainder(x=w698, y=w696) -> (x-y*floor(x/y)=w697:i32)  [unwired: 1 out]
        n336 = Build Array (concatenate)(w716, w715) -> (w714:timestamp[])
        n337 = Build Array (concatenate)(w693, w689) -> (w724:dbl[])
        n338 = Build Array (concatenate)(w692, w690) -> (w722:dbl[])
        n339 = Equal?(x=w697, y=w695) -> (x = y?=w702:bool)
        n340 = Bundle By Name(cluster=w723, "Stats.TRA Position X"=w724, "Stats.TRA PositionY"=w722, "Stats.Stat Centriod X"=w721, "Stats.Stat Centriod Y"=w699, "Stats.Time"=w714) -> (w713:T19)
        n341 = case shown="True" w702 {
          tunnel: w701 -> [w759 w762]
          tunnel: [w759 w760] -> w700
          frame False {
          }
          frame True {
            n342 = call <vilib>:"Add State(s) to Queue__jki_lib_state_machine.vi"("State(s) in (\"\")"=w762, "State(s) at Back (\"\")"="Save Stats" ("State(s) at Back (\"\")")) -> ("States Out"=w760:string)  [unwired: 13 in]
          }
        }
        n343 = Unbundle By Name(w713) -> ("Stats.Time"=w709:timestamp[], "Stats.Stat Centriod X"=w712:dbl[], "Stats.Stat Centriod Y"=w711:dbl[], "Stats.TRA Position X"=w710:dbl[], "Stats.TRA PositionY"=w708:dbl[])
        n344 = call <vilib>:"Add State(s) to Queue__jki_lib_state_machine.vi"("State(s) in (\"\")"=w700) -> ("States Out"=w726:string)  [unwired: 14 in]
        n345 = Bundle("Time"=w709, "Stat Centriod X"=w712) -> (w707:T22)  [unwired: 1 in]
        n346 = Bundle("Time"=w709, "Stat Centriod Y"=w711) -> (w706:T23)  [unwired: 1 in]
        n347 = Bundle("Time"=w709, "TRA Position X"=w710) -> (w705:T24)  [unwired: 1 in]
        n348 = Bundle("Time"=w709, "TRA PositionY"=w708) -> (w704:T25)  [unwired: 1 in]
        n349 = Build Array(w707, w706, w705, w704) -> (→"Stats":T26)
      }
      frame "Calibrate" {
        # "Your code here.\n(You can make a copy of, or modify, this frame)"
        n350 = Unbundle By Name(w774) -> ("RelativeMove.Axis 1.CW::2"=w767:refnum<vi>, "RelativeMove.Axis 1.CCW::2"=w766:refnum<vi>)
        n351 = control-ref of="RelativeSettings.Axis 1.Position::2"() -> (w765:refnum<vi>)
        n352 = Unbundle By Name(w773) -> ("beam detection para"=w769:T3)
        n353 = Decimal String To Number(string=w771) -> (number=w768:i32)  [unwired: 2 in, 1 out]
        n354 = Build Array(w765, w765) -> (w764:refnum<vi>[])
        n355 = Build Array(w767, w766) -> (w763:refnum<vi>[])
        n356 = call "CalibrateSingleAxis.vi"("Numeric"=w768, "beam detection para"=w769, "error in (no error)"=w772, "RelativeSettings.Axis 1"=w764, "RelativeMove.Axis 1"=w763, "Refnum in"=w770) -> ()  [unwired: 2 in, 4 out]
        n357 = call <vilib>:"Add State(s) to Queue__jki_lib_state_machine.vi"("State(s) in (\"\")"=w776) -> ("States Out"=w775:string)  [unwired: 14 in]
      }
      frame "New Category: 2" {
        # "Your code here.\n(You can make a copy of, or modify, this frame)"
        n358 = call <vilib>:"Add State(s) to Queue__jki_lib_state_machine.vi"("State(s) in (\"\")"=w780) -> ("States Out"=w779:string)  [unwired: 14 in]
      }
    }
    n359 = disable-structure shown="Disabled" {
      disable-tunnel: "ActiveMotorName::2" -> [w53 _]
      disable-tunnel: "ActiveMotor" -> [w50 _]
      frame Disabled {
        n360 = property on="ActiveMotor" class="Ring (strict)"() -> ("Strings []"=w49:string[])  [unwired: 2 in, 2 out]
        n361 = Index Array(array=w49, index=w50) -> (element=w51:string)
        n362 = Not Equal?(x=w53, y=w51) -> (x != y?=w52:bool)
        n363 = case shown="True" w52 {
          tunnel: w49 -> [_ w56]
          tunnel: w53 -> [_ w55]
          frame False {
          }
          frame True {
            n364 = Search 1D Array(1D array=w56, element=w55) -> (index of element=w54:i32)  [unwired: 1 in]
            n365 = property on="ActiveMotor" class="Ring (strict)"("Value"=w54) -> ()  [unwired: 2 in, 2 out]
          }
        }
      }
      frame Enabled {
      }
    }
  }
  n366 = control-ref of="This Application"() -> (w11:refnum<vi>)
  n367 = control-ref of="This VI"() -> (w15:refnum<vi>)
  n368 = Current VI's Menubar() -> (w14:refnum<k9>)
  n369 = call "supergui create stop queue.vi"() -> ("STOP Queue out"=w1:refnum<queue>)  [unwired: 11 in]
  n370 = call "GUI_Master_subvi_reentrant_queues.vi"("STOP Queue in"=w1, "This Application"=w11, "error in (no error)"=w12, "tcp data event"=w10, "Caller menu reference"=w14, "Caller VI ref"=w15) -> ("error out"=w23:errorcluster)  [unwired: 5 in]
  n371 = call <vilib>:"Clear Errors.vi"("error in (no error)"=w23) -> ("error out"=w21:errorcluster)  [unwired: 6 in]
  n372 = call "IMAQ Dispose"("error in (no error)"=w21) -> ("error out"=w20:errorcluster)  [unwired: 5 in]
  n373 = call "IMAQ Dispose"("Image"=w16, "error in (no error)"=w20) -> ("error out"=→"error IO 2":errorcluster)  [unwired: 4 in]
